vi "GTcode_v7.vi"() -> ()   [LabVIEW 2016]
uses:
  flex05-4chPascal.dll
  <vilib>/Utility/config.llb/NI_LVConfig.lvlib
  <vilib>/Utility/config.llb/Write Key (U32).vi
  <vilib>/Utility/config.llb/Read Key (U32).vi
  flex05oem8chauto100nsPASCAL_win7.dll
  <vilib>/Analysis/NI_AALBase.lvlib
  <vilib>/Utility/config.llb/Write Key (Double).vi
  <vilib>/Utility/config.llb/Read Key (I32).vi
  <vilib>/Utility/config.llb/Write Key (String).vi
  <vilib>/Utility/config.llb/Write Key (I32).vi
panel:
  out "EMG Value Text":string
  out "display number":dbl
  in  "Tab Control":T1(tab)=enum."Real Time Fitting Parameters"
  out "EMG":dbl(slide) scale=0.0..100.0
  out "mean":dbl format="%0.1e"
  out "COV":dbl format="%0.1f"
  in  "Fixed Time":bool
  in  "Detector Used":T2(ring)=enum."Det 2"
  in  "Real Time Fitting?":bool=TRUE
  out "g2":cluster{"Delay Time":sgl[], sgl[]}[](graph) caption="Normalized Correlation Function"
  out "Tau":cluster{"tmp":dbl, dbl}(graph) caption="Relative Changes of Flow"
  in  "QUIT":bool
  in  "Clear plots":bool
  in  "Baseline":bool
  in  "MARK\nMark":bool
  in  "Stop":bool
  out "Mark #":u32
  out "Trial #":u32
  out "Frame #":u32
  out "Det 8":sgl format="%.3f"
  out "Det 7":sgl format="%.3f"
  out "Det 6":sgl format="%.3f"
  out "Det 5":sgl format="%.3f"
  out "Det 4":sgl format="%.3f"
  out "Det 3":sgl format="%.3f"
  out "Det 2":sgl format="%.3f"
  out "Det 1":sgl format="%.3f"
  out "Computer Time":string="2010-1-12 23:16:10"
  in  "D1":bool
  in  "D2":bool
  in  "D3":bool
  in  "D4":bool
  in  "D5":bool
  in  "D6":bool
  in  "D7":bool
  in  "D8":bool
  out "Tau 2":T3(graph)={1.6593152555505744e-08, 3.9427894777554196e-08, 4.065716407938411e-08, 1.5135790977358522e-08, 2.4870420100428357e-08, 7.094765128107397e-08, 0.0, 4.1348620928852906e-07, 1.5886917674344795e-08, 4.0280526032721455e-08, -1.0, -1.0} caption="Blood Flow Index (cm2/s)"
  in  "Fixed # of Frames":u32=5
  out "Status":string="Quit"
  in  "Optical Switch OPEN":bool
  in  "Delay between frames(ms)":u32=500
  out "Time Left (ms)":sgl format="%.3f"
  in  "Integration Time (ms)":sgl=1000.0 min=1 max=13000 step=1
  in  "File Name (mouse#):":string="test0"
  in  "Data Save Directory:":path=path "C:/data"
  in  "ISS Lasers ON":bool
  in  "Test":bool
  in  "Right":bool
  out "R Counter":dbl format="%#_13g"
  out "saved file name":string
  in  "Left":bool
  out "L Counter":dbl format="%#_13g"
  in  "Lines":tag="Dev1/port1/line0:1, Dev1/port1/line3:7"
  in  "Delaytime(ms)":u32=200
  in  "Initialize Correlator":bool
  in  "Detector Select":enum32{"4 Detectors", "8 Detectors"}(radio)=enum."8 Detectors"
  in  "Update Time (ms)\nDO NOT CHANGE!":u32=105 min=1 max=999 step=1
  in  "Laser Input Name":refnum<visa-resource-name>="COM7"
  out "Change?":bool
  in  "Sequence Scan":bool
  out "Flow in each detector":dbl[](array[numeric])=[-1.0, -1.0, -1.0, -1.0, -1.0, -1.0, -1.0, -1.0, -1.0, -1.0, -1.0, -1.0]
  in  "Visible Averages":bool[](array[boolean])=[FALSE, FALSE, FALSE, FALSE]
  in  "Avg":bool[][](array[boolean])=[[FALSE, FALSE, FALSE, FALSE, FALSE, FALSE, FALSE, FALSE], [FALSE, FALSE, FALSE, FALSE, FALSE, FALSE, FALSE, FALSE], [FALSE, FALSE, FALSE, FALSE, FALSE, FALSE, FALSE, FALSE], [FALSE, FALSE, FALSE, FALSE, FALSE, FALSE, FALSE, FALSE]]
  in  "rho":dbl[](array[numeric])=[2.5, 2.5, 2.5, 2.5, 2.5, 2.5, 2.5, 2.5, -1.0, -1.0, -1.0, -1.0]
  in  "Other Settings":u32[](array[numeric])=[1, 120, 0, 1] caption="Flow in each detector"
  in  "Initial Guess":dbl[](array[numeric])=[1e-08, 0.5, 0.05, 10.0] caption="Flow in each detector"
  in  "UI Data Path":path=path "C:/Users/Tinggroup/Desktop/VRMuscleActivationVisualizer/LabviewFiles/Jake DCScode_GT/BiofeedbackEMGPackage/BiofeedbackData.txt"
  in  "FPS":dbl
  out "4CH?":bool
  out "Detector#":u32=1
  out "Source#":u32=1
  # "kHz"
  # "kHz"
  # "Don't Change these Parameters unless you know clearly what you are doing"
  # "ISS Triggers Setup"
  # "Channel Parameters"
  # "Step1"
  # "Line"
  # "0"
  # "1"
  # "3"
  # "4"
  # "5"
  # "6"
  # "7"
  # "*The number of lines in the list must\nmatch the number of elements in\nthe array."
  # "Step2"
  # "Line"
  # "0"
  # "1"
  # "3"
  # "4"
  # "5"
  # "6"
  # "7"
  # "Step3"
  # "Line"
  # "0"
  # "1"
  # "3"
  # "4"
  # "5"
  # "6"
  # "7"
  # "Line    Signal\n\n0           ISS Trigger (0: OFF, 1: ON)\n1           Flow Laser 1 ON/OFF (0:OFF, 1:ON)\n2           ISS Data Acquisition (0: DONE, 1: NO)\n3           ISS Laser ON/OFF (0: ON, 1: OFF)\n4           Trigger for Marks  (0: OFF, 1: ON)\n5           Flow Laser 2 ON/OFF (0:OFF, 1:ON)\n6           Reserved\n7           Reserved"
  # "Wait ISS Data Acuisition DONE Signal"
  # "Step4"
  # "Step5"
  # "Line"
  # "0"
  # "1"
  # "3"
  # "4"
  # "5"
  # "6"
  # "7"
  # "Flow Lasers Setup"
  # "FROM FRONT PANEL"
  # "Line"
  # "0"
  # "1"
  # "3"
  # "4"
  # "5"
  # "6"
  # "7"
  # "Line"
  # "0"
  # "1"
  # "3"
  # "4"
  # "5"
  # "6"
  # "7"
  # "Det 1"
  # "Det 2"
  # "Det 3"
  # "Det 4"
  # "Det 5"
  # "Det 6"
  # "Det 7"
  # "Det 8"
  # "Avg 1"
  # "Avg 2"
  # "Avg 3"
  # "Avg 4"
  # "Db"
  # "Beta"
  # "Mua"
  # "MuS'"
  # "1"
  # "2"
  # "3"
  # "4"
  # "5"
  # "6"
  # "7"
  # "8"
  # "Avg 1"
  # "Starting Pt"
  # "End Pt"
  # "Approximate"
  # "Variables"
  # "Avg 2"
  # "Avg 3"
  # "Avg 4"
  # "Source Detector  Separations"
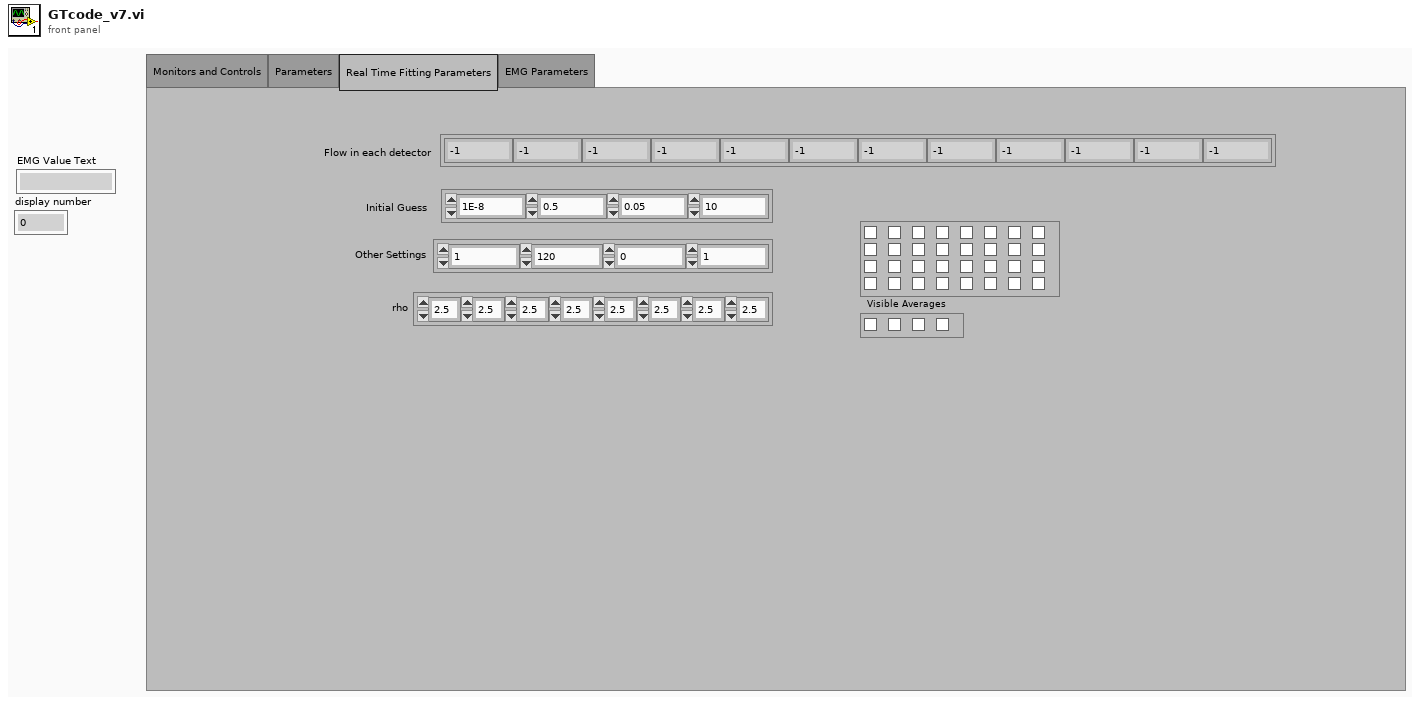
[diagram p1: front panel]
types:
  T1 = enum32{"Monitors and Controls", "Parameters", "Real Time Fitting Parameters", "EMG Parameters"}
  T2 = enum16{"Det 1", "Det 2", "Det 3", "Det 4", "Det 5", "Det 6", "Det 7", "Det 8"}
  T3 = cluster{dbl, dbl, dbl, dbl, dbl, dbl, dbl, dbl, dbl, dbl, dbl, dbl}
  T4 = enum8{"Enabled", "Disabled", "Disabled and Grayed Out"}
  T5 = cluster{dbl, dbl, dbl, dbl, dbl, dbl, dbl, dbl, dbl, dbl, dbl, dbl}[]
  T6 = typedef "NI_LVConfig.lvlib/Config Data RefNum.ctl" = refnum<k1>
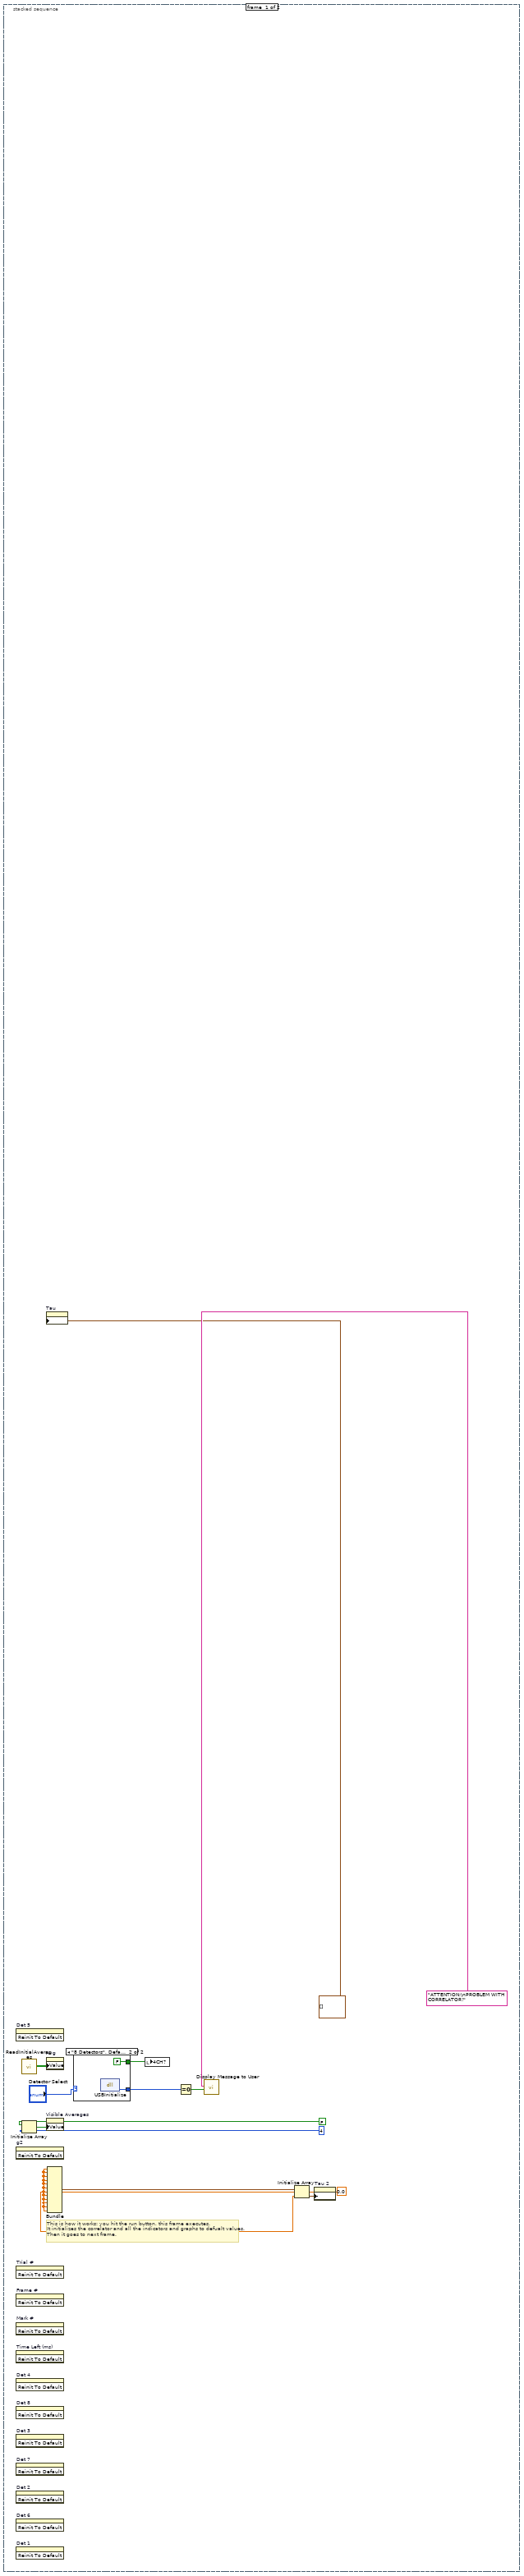
[diagram p2: hidden frame]
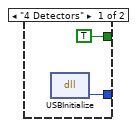
[diagram p3: hidden frame]
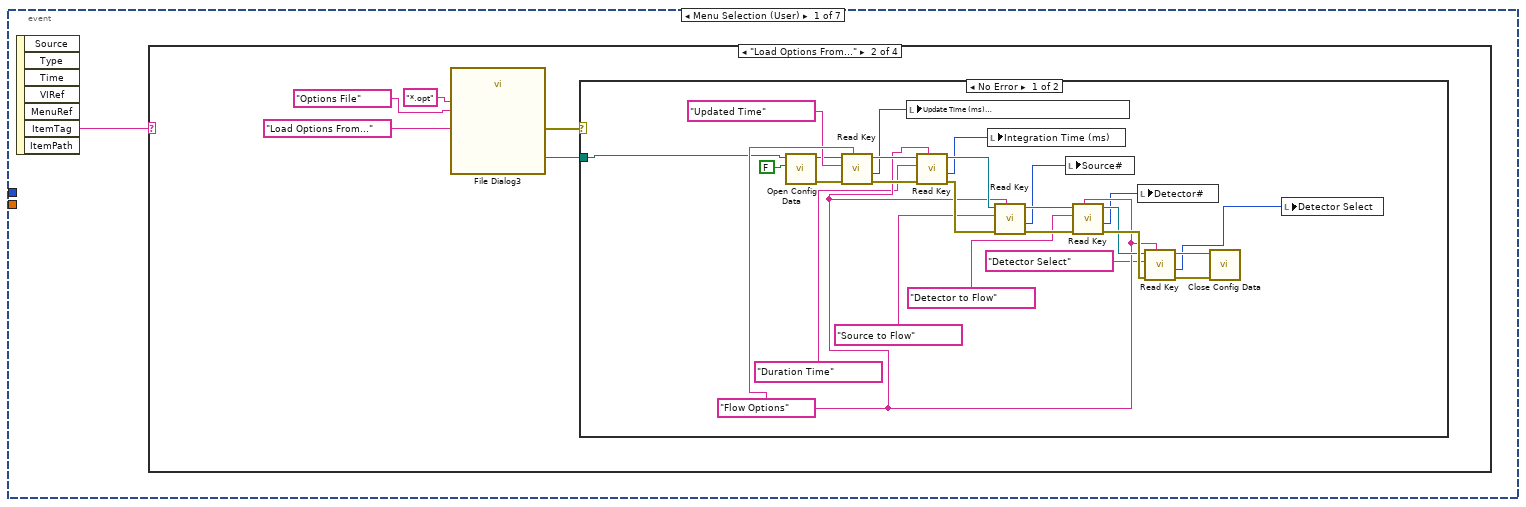
[diagram p5: hidden frame]
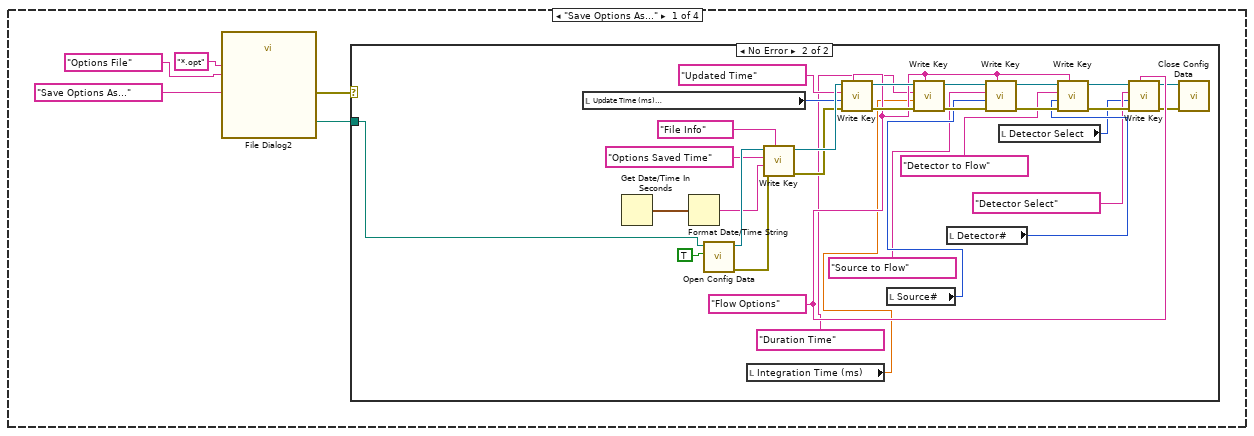
[diagram p6: hidden frame]
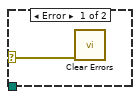
[diagram p7: hidden frame]
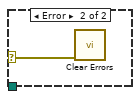
[diagram p8: hidden frame]
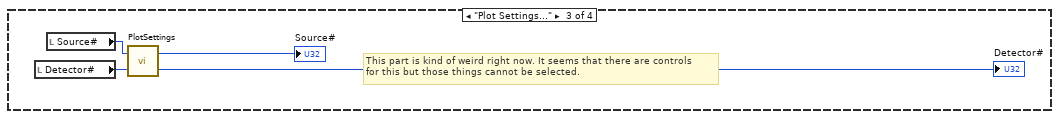
[diagram p9: hidden frame]
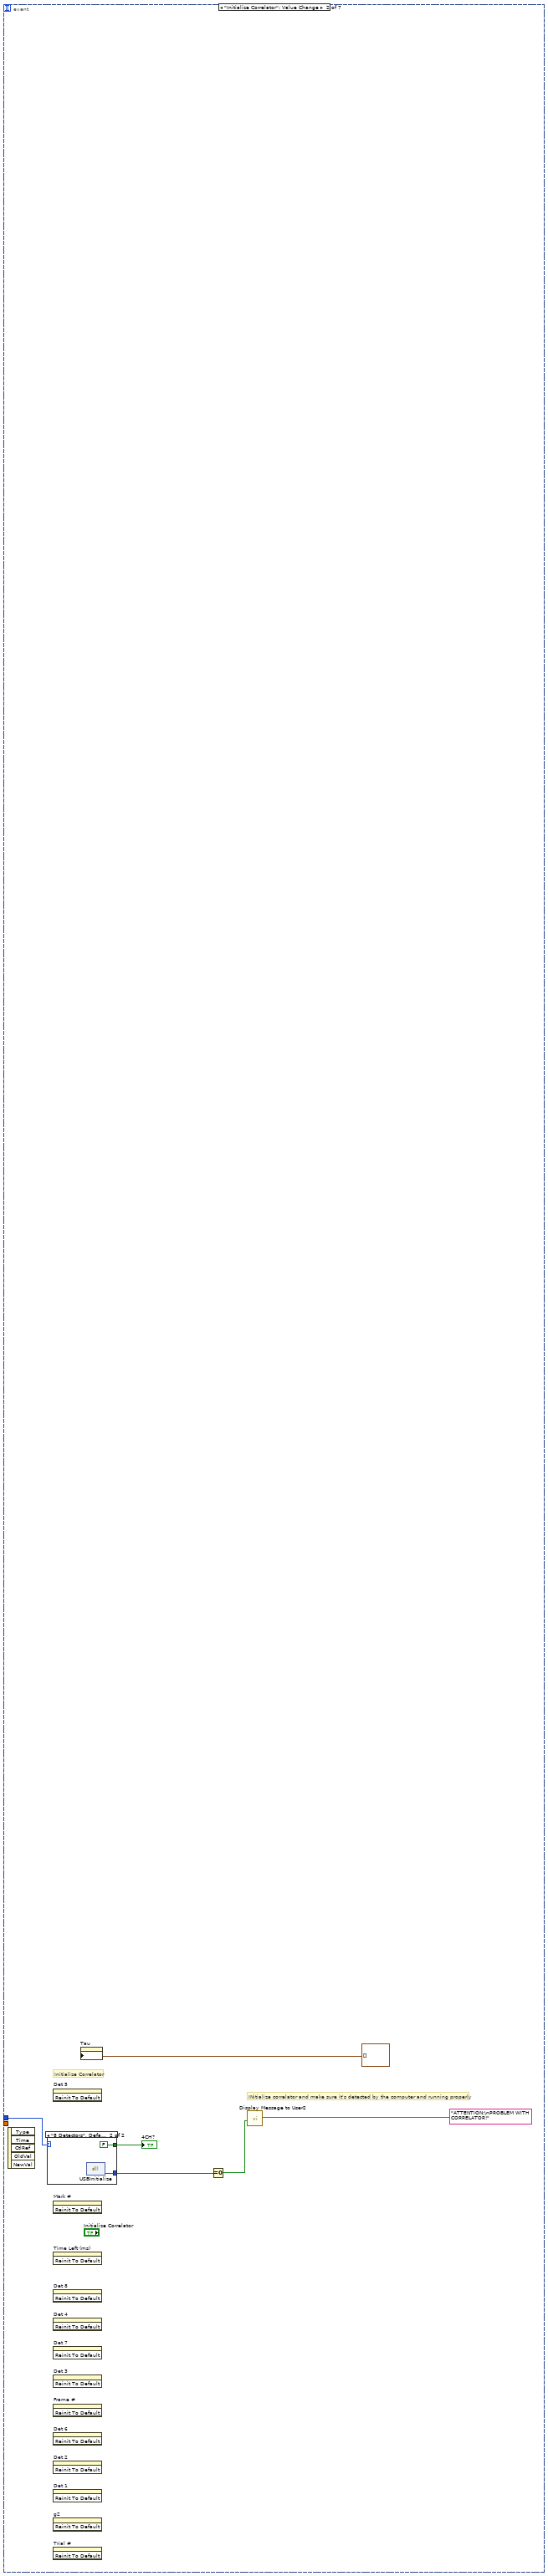
[diagram p11: hidden frame]
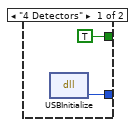
[diagram p12: hidden frame]
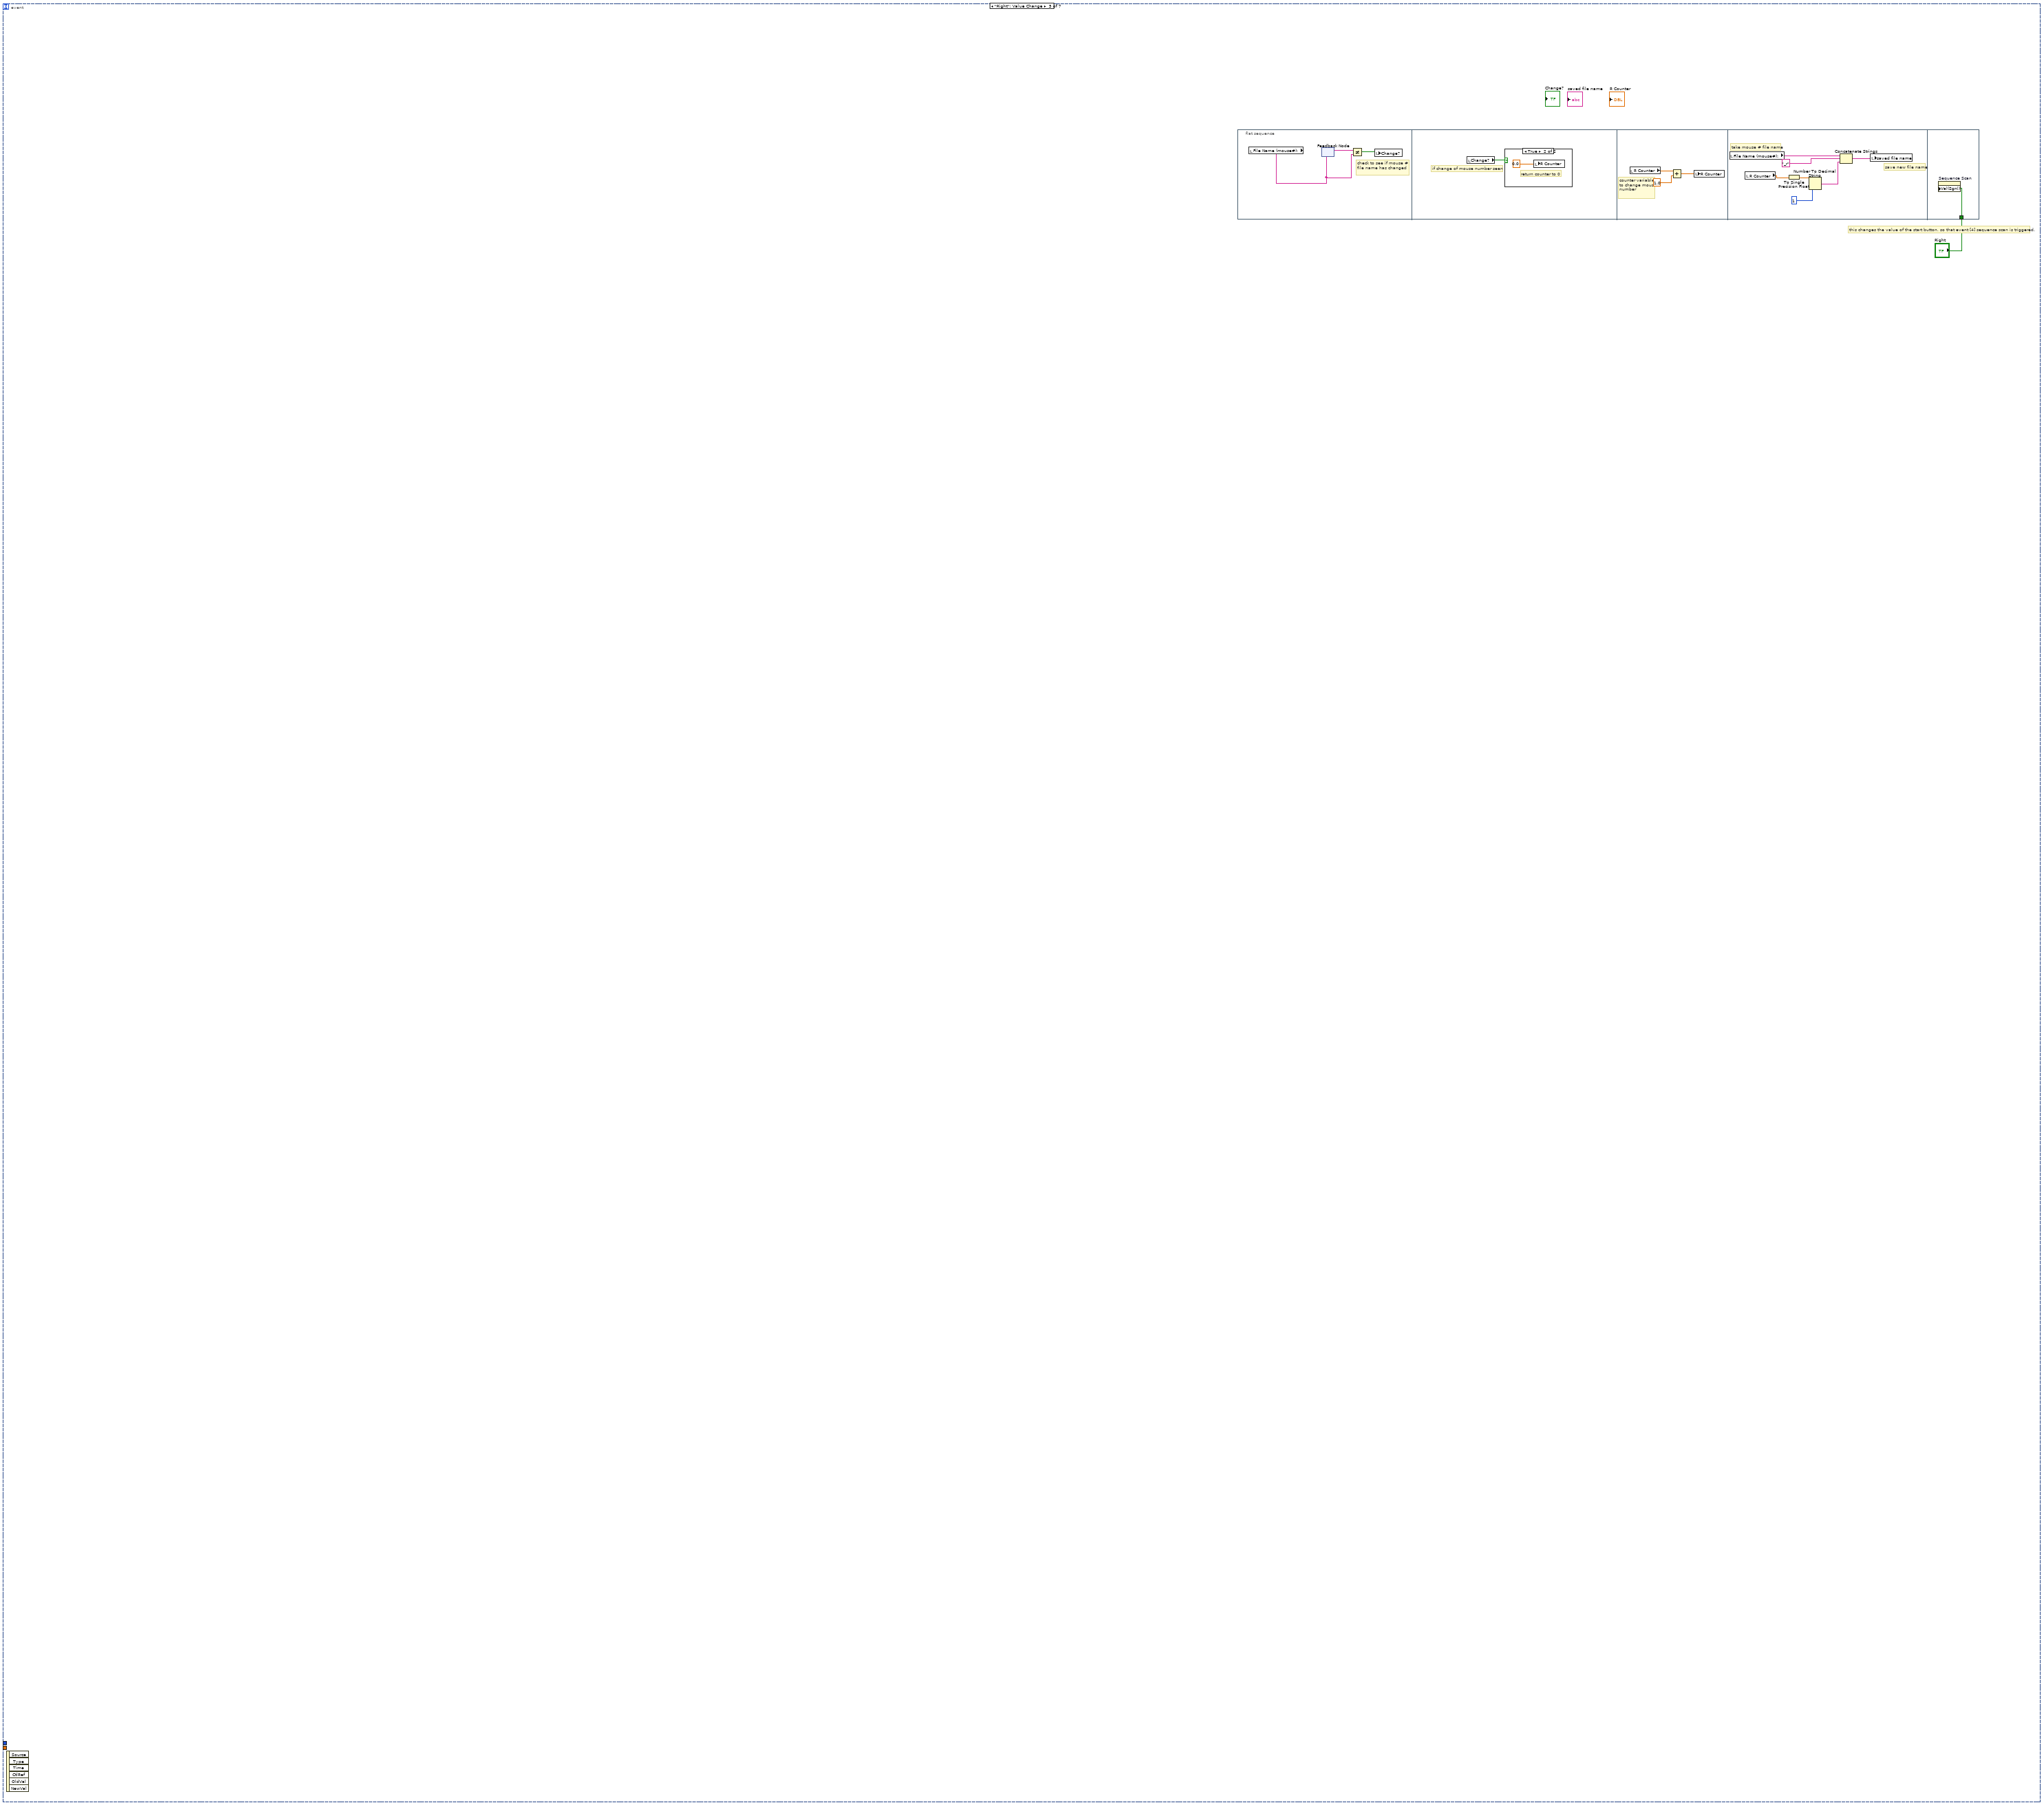
[diagram p13: hidden frame]
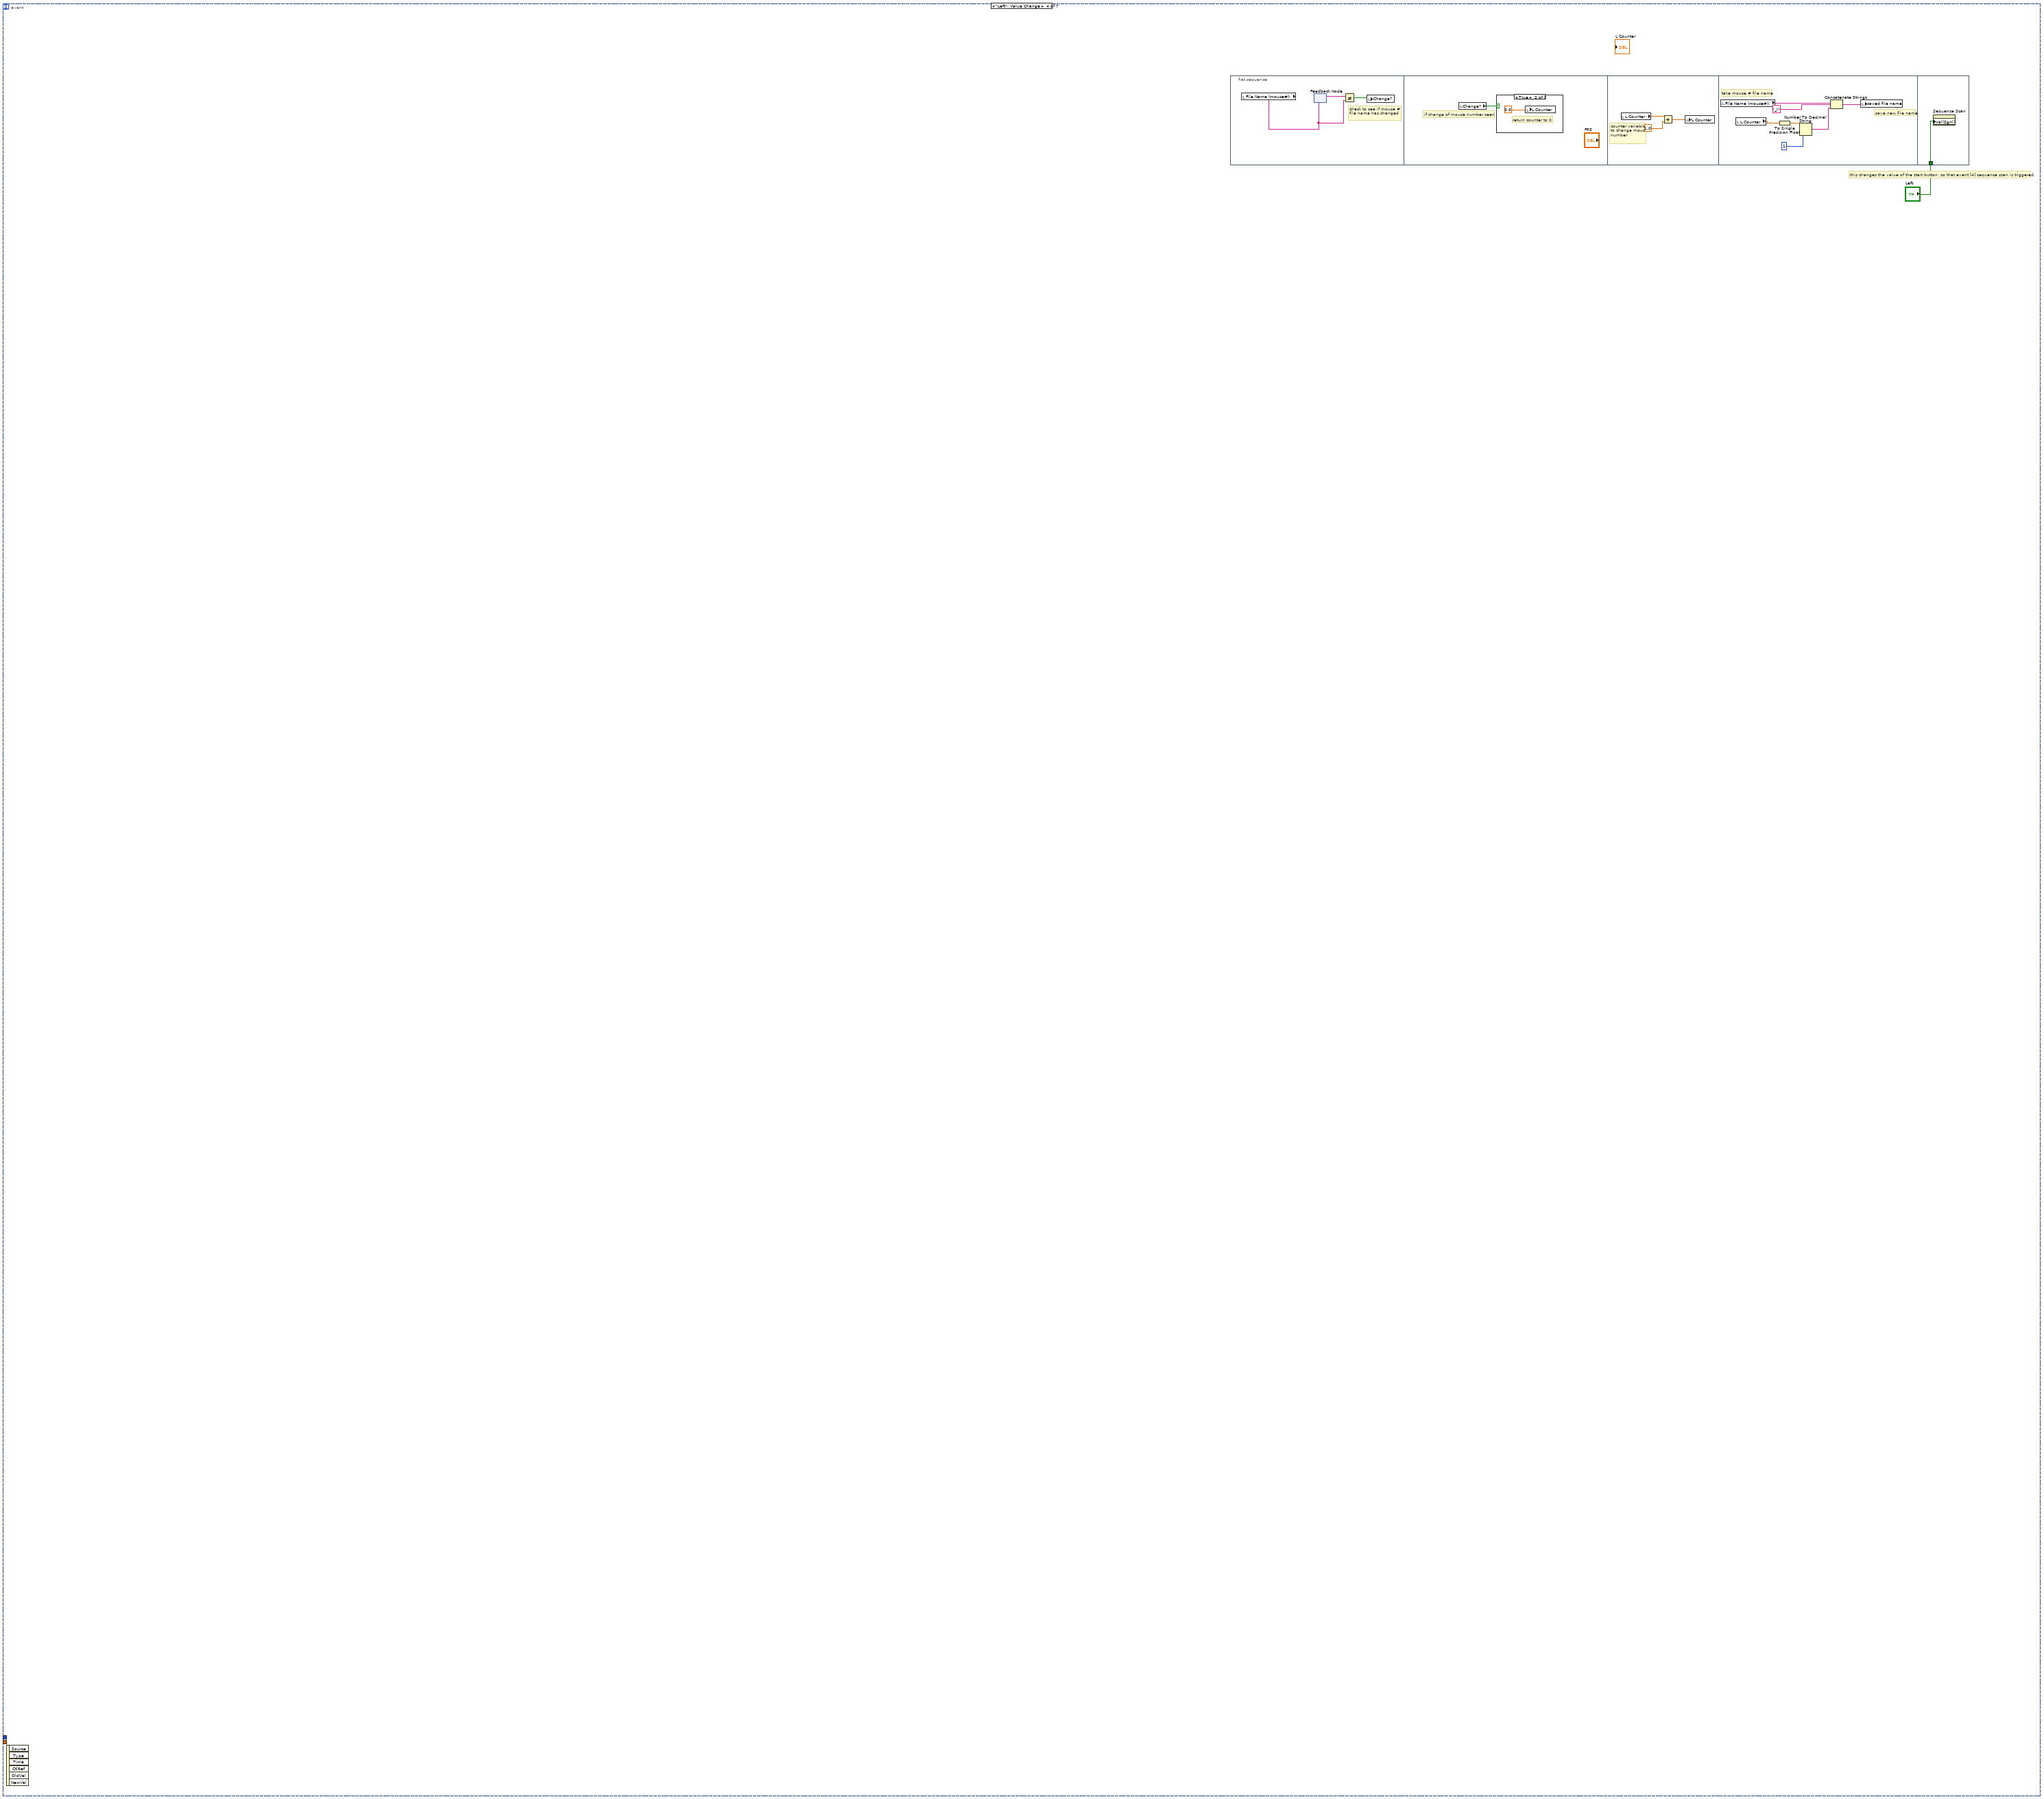
[diagram p15: hidden frame]
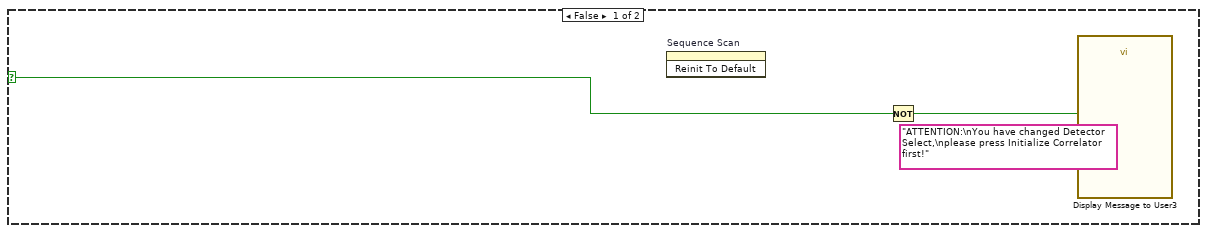
[diagram p17: hidden frame]
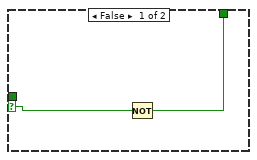
[diagram p18: hidden frame]
diagram:
  n1 = while {
    stop <- w6 stop-if-true
    n2 = local read "UI Data Path"() -> (w7:path)
    n3 = local read "Stop"() -> (w6:bool)
    n4 = Read from Text File(file (use dialog)=w7) -> (text=w5:string)  [unwired: 3 in, 3 out]
    "EMG Value Text" <- w5
    n5 = Fract/Exp String To Number(string=w5) -> (number=→"display number" →"EMG":dbl)  [unwired: 3 in, 1 out]
  }
  n6 = local read "Laser Input Name"() -> (w2:refnum<visa-resource-name>)
  n7 = call "BioFeedback7(DAQ+8-channel)SubVIToUI.vi"("UI Data Input File"="UI Data Path") -> ()  [unwired: 15 in]
  n8 = call "iBs.vi"("Laser On/Off"=FALSE, "VISA resource name"=w2) -> ()
  n9 = stacked-sequence {
    frame #0 {
      w10 = 0.0
      # "This is how it works: you hit the run button, this frame executes.\nIt initializes the correlator and all the indicators and graphs to defualt values.\nThen it goes to next frame."
      n10 = invoke on="Det 5" class="DigNum (strict)" method="Reinit To Default"() -> ()  [unwired: 3 in, 3 out]
      n11 = invoke on="g2" class="XYGraph (strict)" method="Reinit To Default"() -> ()  [unwired: 3 in, 3 out]
      n12 = invoke on="Trial #" class="DigNum (strict)" method="Reinit To Default"() -> ()  [unwired: 3 in, 3 out]
      n13 = invoke on="Frame #" class="DigNum (strict)" method="Reinit To Default"() -> ()  [unwired: 3 in, 3 out]
      n14 = invoke on="Mark #" class="DigNum (strict)" method="Reinit To Default"() -> ()  [unwired: 3 in, 3 out]
      n15 = invoke on="Time Left (ms)" class="DigNum (strict)" method="Reinit To Default"() -> ()  [unwired: 3 in, 3 out]
      n16 = invoke on="Det 4" class="DigNum (strict)" method="Reinit To Default"() -> ()  [unwired: 3 in, 3 out]
      n17 = invoke on="Det 8" class="DigNum (strict)" method="Reinit To Default"() -> ()  [unwired: 3 in, 3 out]
      n18 = invoke on="Det 3" class="DigNum (strict)" method="Reinit To Default"() -> ()  [unwired: 3 in, 3 out]
      n19 = invoke on="Det 7" class="DigNum (strict)" method="Reinit To Default"() -> ()  [unwired: 3 in, 3 out]
      n20 = invoke on="Det 2" class="DigNum (strict)" method="Reinit To Default"() -> ()  [unwired: 3 in, 3 out]
      n21 = invoke on="Det 6" class="DigNum (strict)" method="Reinit To Default"() -> ()  [unwired: 3 in, 3 out]
      n22 = invoke on="Det 1" class="DigNum (strict)" method="Reinit To Default"() -> ()  [unwired: 3 in, 3 out]
      n23 = call "ReadInitialAverages.vi"() -> ("avgOut"=w9:bool[][])  [unwired: 11 in]
      n24 = Initialize Array(FALSE, 4) -> (w8:bool[])
      n25 = property on="Tau" class="WFChart (strict)"("History Data"=cluster{"tmp":dbl, dbl}[] []) -> ()  [unwired: 2 in, 2 out]
      n26 = property on="Avg" class="Arr (strict)"("Value"=w9) -> ()  [unwired: 2 in, 2 out]
      n27 = property on="Visible Averages" class="Arr (strict)"("Value"=w8) -> ()  [unwired: 2 in, 2 out]
      n28 = Bundle(w10, w10, w10, w10, w10, w10, w10, w10, w10, w10, w10, w10) -> (w12:T3)  [unwired: 1 in]
      n29 = case shown="\"8 Detectors\", Default" "Detector Select" {
        tunnel: [w22 w24] -> w20
        tunnel: [TRUE FALSE] -> w18
        frame "4 Detectors" {
          n30 = dll-call lib="C:/Users/BUCKLEY-ADMIN/Desktop/GTcode_v6_Michelle/flex05-4chPascal.dll" fn="USBInitialize" label="InitCH4"() -> ("return type"=w22:u8)  [unwired: 3 in, 2 out]
        }
        frame "8 Detectors", Default {
          n31 = dll-call lib="C:/Users/BUCKLEY-ADMIN/Desktop/GTcode_v6_Michelle/flex05oem8chauto100nsPASCAL_win7.dll" fn="USBInitialize" label="InitCH8"() -> ("return type"=w24:u8)  [unwired: 3 in, 2 out]
        }
      }
      n32 = local write "4CH?"(w18) -> ()
      n33 = Equal To 0?(x=w20) -> (x = 0?=w19:bool)
      n34 = call "Display Message to User"("Enable"=w19, "Message"="ATTENTION:\nPROBLEM WITH CORRELATOR!") -> ()  [unwired: 8 in, 2 out]
      n35 = Initialize Array(w12, w10) -> (w11:T5)
      n36 = property on="Tau 2" class="WFChart (strict)"("History Data"=w11) -> ()  [unwired: 2 in, 2 out]
    }
    frame #1 {
      n37 = while {
        stop <- w28 stop-if-true
        # "Looks at whether using 4 or 8 ch correlator\nGenerates time points for g2 function based on correlator"
        n38 = local read "Detector Select"() -> (w26:enum32{"4 Detectors", "8 Detectors"})
        n39 = case shown="\"8 Detectors\"" w26 {
          tunnel: [_ w29] -> w25
          frame "4 Detectors", Default {
          }
          frame "8 Detectors" {
            n40 = formula code="int i,j;\nfloat DelayTime[256];\nfloat first_delay;\n\nfirst_delay = 2E-7;\n\nfor(i=0;i<16;i++)\nDelayTime[i] = (i+1)*first_delay;\nfor(j=1;j<31;j++)\n    for(i=0;i<8;i++)\n         DelayTime[i+(j-1)*8+16] = DelayTime[(j-1)*8+16+i-1]+first_delay*pow(2,j);"() -> ("DelayTime"=w29:dbl[])
          }
        }
        n41 = event shown="[4] \"Sequence Scan\": Value Change" {
          selector: _ -> [_ _ _ _ _ _ _]
          dyn-events: _ -> [_ _ _ _ _ _ _]
          timeout: 500 -> [_ _ _ _ _ _ _]
          tunnel: w25 -> [_ _ _ _ w153 _ _]
          tunnel: [_ _ _ _ _ "QUIT" _] -> w28
          tunnel: w26 -> [_ w106 _ _ w149 w637 _]
          event Menu Selection (User) {
            n42 = event-data() -> ("ItemTag"=w30:string)  [unwired: 1 in, 6 out]
            n43 = case shown="\"Load Options From...\"" w30 {
              frame "Save Options As..." {
                n44 = call "File Dialog2"("prompt"="Save Options As...", "pattern (all files)"="*.opt", "pattern label"="Options File") -> ("selected path"=w32:path, "error out"=w31:errorcluster)  [unwired: 9 in, 2 out]
                n45 = case shown="No Error" w31 {
                  selector: w31 -> [w36 _]
                  tunnel: w32 -> [_ w67]
                  frame Error {
                    n46 = call <vilib>:"Clear Errors.vi"("error in (no error)"=w36) -> ()  [unwired: 5 in, 2 out]
                  }
                  frame No Error {
                    w54 = "Flow Options"
                    n47 = local read "Update Time (ms)\nDO NOT CHANGE!"() -> (w47:u32)
                    n48 = Get Date/Time In Seconds() -> (seconds since 1Jan1904=w53:timestamp)
                    n49 = Format Date/Time String(seconds (now)=w53) -> (date/time string=w49:string)  [unwired: 2 in]
                    n50 = call <vilib>:"Open Config Data.vi"("create file if necessary (T)"=TRUE, "configuration file path"=w67) -> ("error out"=w65:errorcluster, "refnum"=w64:T6)  [unwired: 7 in, 1 out]
                    n51 = local read "Integration Time (ms)"() -> (w45:sgl)
                    n52 = call-poly <vilib>:"Write Key.vi"("section"="File Info", "error in (no error)"=w65, "value"=w49, "key"="Options Saved Time", "refnum"=w64) -> ("error out"=w51:errorcluster, "refnum out"=w52:T6)  [unwired: 4 in, 1 out]
                    n53 = call-poly <vilib>:"Write Key.vi"("section"=w54, "error in (no error)"=w51, "value"=w47, "key"="Updated Time", "refnum"=w52) -> ("error out"=w63:errorcluster, "refnum out"=w62:T6)  [unwired: 4 in, 1 out]
                    n54 = local read "Source#"() -> (w44:u32)
                    n55 = call-poly <vilib>:"Write Key.vi"("section"=w54, "error in (no error)"=w63, "value"=w45, "key"="Duration Time", "refnum"=w62) -> ("error out"=w58:errorcluster, "refnum out"=w59:T6)  [unwired: 4 in, 1 out]
                    n56 = local read "Detector#"() -> (w41:u32)
                    n57 = call-poly <vilib>:"Write Key.vi"("section"=w54, "error in (no error)"=w58, "value"=w44, "key"="Source to Flow", "refnum"=w59) -> ("error out"=w60:errorcluster, "refnum out"=w61:T6)  [unwired: 4 in, 1 out]
                    n58 = local read "Detector Select"() -> (w39:enum32{"4 Detectors", "8 Detectors"})
                    n59 = call-poly <vilib>:"Write Key.vi"("section"=w54, "error in (no error)"=w60, "value"=w41, "key"="Detector to Flow", "refnum"=w61) -> ("error out"=w57:errorcluster, "refnum out"=w56:T6)  [unwired: 4 in, 1 out]
                    n60 = call-poly <vilib>:"Write Key.vi"("section"=w54, "error in (no error)"=w57, "value"=w39, "key"="Detector Select", "refnum"=w56) -> ("error out"=w37:errorcluster, "refnum out"=w38:T6)  [unwired: 4 in, 1 out]
                    n61 = call <vilib>:"Close Config Data.vi"("error in (no error)"=w37, "refnum"=w38) -> ()  [unwired: 8 in, 2 out]
                  }
                }
              }
              frame "Load Options From..." {
                n62 = call "File Dialog3"("prompt"="Load Options From...", "pattern (all files)"="*.opt", "pattern label"="Options File") -> ("selected path"=w69:path, "error out"=w68:errorcluster)  [unwired: 9 in, 2 out]
                n63 = case shown="No Error" w68 {
                  selector: w68 -> [_ w98]
                  tunnel: w69 -> [w73 _]
                  frame No Error {
                    w88 = "Flow Options"
                    n64 = call <vilib>:"Open Config Data.vi"("create file if necessary (T)"=FALSE, "configuration file path"=w73) -> ("error out"=w80:errorcluster, "refnum"=w79:T6)  [unwired: 7 in, 1 out]
                    n65 = call-poly <vilib>:"Read Key.vi"("section"=w88, "error in (no error)"=w80, "key"="Updated Time", "refnum"=w79) -> ("error out"=w96:errorcluster, "value"=w78:u32, "refnum out"=w95:T6)  [unwired: 4 in, 1 out]
                    n66 = local write "Update Time (ms)\nDO NOT CHANGE!"(w78) -> ()
                    n67 = call-poly <vilib>:"Read Key.vi"("section"=w88, "error in (no error)"=w96, "key"="Duration Time", "refnum"=w95) -> ("error out"=w91:errorcluster, "value"=w77:i32, "refnum out"=w92:T6)  [unwired: 4 in, 1 out]
                    n68 = local write "Integration Time (ms)"(w77) -> ()
                    n69 = call-poly <vilib>:"Read Key.vi"("section"=w88, "error in (no error)"=w91, "key"="Source to Flow", "refnum"=w92) -> ("error out"=w93:errorcluster, "value"=w74:u32, "refnum out"=w94:T6)  [unwired: 4 in, 1 out]
                    n70 = local write "Source#"(w74) -> ()
                    n71 = call-poly <vilib>:"Read Key.vi"("section"=w88, "error in (no error)"=w93, "key"="Detector to Flow", "refnum"=w94) -> ("error out"=w90:errorcluster, "value"=w75:u32, "refnum out"=w89:T6)  [unwired: 4 in, 1 out]
                    n72 = local write "Detector#"(w75) -> ()
                    n73 = call-poly <vilib>:"Read Key.vi"("section"=w88, "error in (no error)"=w90, "key"="Detector Select", "refnum"=w89) -> ("error out"=w81:errorcluster, "value"=w76:u32, "refnum out"=w82:T6)  [unwired: 4 in, 1 out]
                    n74 = call <vilib>:"Close Config Data.vi"("error in (no error)"=w81, "refnum"=w82) -> ()  [unwired: 8 in, 2 out]
                    n75 = local write "Detector Select"(w76) -> ()
                  }
                  frame Error {
                    n76 = call <vilib>:"Clear Errors.vi"("error in (no error)"=w98) -> ()  [unwired: 5 in, 2 out]
                  }
                }
              }
              frame "Plot Settings..." {
                # "This part is kind of weird right now. It seems that there are controls\nfor this but those things cannot be selected."
                n77 = local read "Detector#"() -> (w100:u32)
                n78 = local read "Source#"() -> (w101:u32)
                n79 = call "PlotSettings.vi"("Detectorin"=w100, "Sourcein"=w101) -> ("Detector#"=→"Detector#":u32, "Source#"=→"Source#":u32)
              }
              frame Default {
              }
            }
          }
          event "Initialize Correlator": Value Change {
            # "INitialize correlator and make sure it's detected by the computer and running properly"
            # "Initialize Correlator"
            n80 = event-data() -> ()  [unwired: 1 in, 5 out]
            n81 = case shown="\"8 Detectors\", Default" w106 {
              tunnel: [w110 w112] -> w108
              tunnel: [TRUE FALSE] -> w105
              frame "4 Detectors" {
                n82 = dll-call lib="C:/Users/BUCKLEY-ADMIN/Desktop/GTcode_v6_Michelle/flex05-4chPascal.dll" fn="USBInitialize" label="InitCH4"() -> ("return type"=w110:u8)  [unwired: 3 in, 2 out]
              }
              frame "8 Detectors", Default {
                n83 = dll-call lib="C:/Users/BUCKLEY-ADMIN/Desktop/GTcode_v6_Michelle/flex05oem8chauto100nsPASCAL_win7.dll" fn="USBInitialize" label="InitCH8"() -> ("return type"=w112:u8)  [unwired: 3 in, 2 out]
              }
            }
            "4CH?" <- w105
            n84 = invoke on="Det 5" class="DigNum (strict)" method="Reinit To Default"() -> ()  [unwired: 3 in, 3 out]
            n85 = invoke on="Mark #" class="DigNum (strict)" method="Reinit To Default"() -> ()  [unwired: 3 in, 3 out]
            n86 = invoke on="Time Left (ms)" class="DigNum (strict)" method="Reinit To Default"() -> ()  [unwired: 3 in, 3 out]
            n87 = invoke on="Det 8" class="DigNum (strict)" method="Reinit To Default"() -> ()  [unwired: 3 in, 3 out]
            n88 = invoke on="Det 4" class="DigNum (strict)" method="Reinit To Default"() -> ()  [unwired: 3 in, 3 out]
            n89 = invoke on="Det 7" class="DigNum (strict)" method="Reinit To Default"() -> ()  [unwired: 3 in, 3 out]
            n90 = invoke on="Det 3" class="DigNum (strict)" method="Reinit To Default"() -> ()  [unwired: 3 in, 3 out]
            n91 = invoke on="Frame #" class="DigNum (strict)" method="Reinit To Default"() -> ()  [unwired: 3 in, 3 out]
            n92 = invoke on="Det 6" class="DigNum (strict)" method="Reinit To Default"() -> ()  [unwired: 3 in, 3 out]
            n93 = invoke on="Det 2" class="DigNum (strict)" method="Reinit To Default"() -> ()  [unwired: 3 in, 3 out]
            n94 = invoke on="Det 1" class="DigNum (strict)" method="Reinit To Default"() -> ()  [unwired: 3 in, 3 out]
            n95 = invoke on="g2" class="XYGraph (strict)" method="Reinit To Default"() -> ()  [unwired: 3 in, 3 out]
            n96 = invoke on="Trial #" class="DigNum (strict)" method="Reinit To Default"() -> ()  [unwired: 3 in, 3 out]
            n97 = property on="Tau" class="WFChart (strict)"("History Data"=cluster{"tmp":dbl, dbl}[] []) -> ()  [unwired: 2 in, 2 out]
            n98 = Equal To 0?(x=w108) -> (x = 0?=w107:bool)
            n99 = call "Display Message to User2"("Enable"=w107, "Message"="ATTENTION:\nPROBLEM WITH CORRELATOR!") -> ()  [unwired: 8 in, 2 out]
          }
          event "Right": Value Change {
            # "this changes the value of the start button, so that event [4] sequence scan is triggered."
            n100 = event-data() -> ()  [unwired: 1 in, 6 out]
            n101 = flat-sequence {
              tunnel: "Right" -> [w129]
              frame #0 {
                # "check to see if mouse # file name has changed"
                n102 = local read "File Name (mouse#):"() -> (w115:string)
                n103 = feedback #1() -> (w116:string)  [unwired: 1 in]
                n104 = feedback-in #1(w115) -> ()
                n105 = Not Equal?(x=w116, y=w115) -> (x != y?=w114:bool)
                n106 = local write "Change?"(w114) -> ()
              }
              frame #1 {
                # "if change of mouse number seen"
                n107 = local read "Change?"() -> (w117:bool)
                n108 = case shown="True" w117 {
                  frame False {
                  }
                  frame True {
                    # "return counter to 0"
                    n109 = local write "R Counter"(0.0) -> ()
                  }
                }
              }
              frame #2 {
                # "counter variable to change mouse number"
                n110 = local read "R Counter"() -> (w120:dbl)
                n111 = Add(x=w120, y=1.0) -> (x+y=w119:dbl)
                n112 = local write "R Counter"(w119) -> ()
              }
              frame #3 {
                # "save new file name"
                # "take mouse # file name"
                n113 = local read "File Name (mouse#):"() -> (w127:string)
                n114 = local read "R Counter"() -> (w122:dbl)
                n115 = To Single Precision Float(number=w122) -> (single precision float=w123:sgl)
                n116 = Number To Decimal String(number=w123, width (-)=1) -> (decimal integer string=w125:string)
                n117 = Concatenate Strings(w127, "_r", w125) -> (w126:string)
                n118 = local write "saved file name"(w126) -> ()
              }
              frame #4 {
                n119 = property on="Sequence Scan" class="Bool (strict)"("Val(Sgnl)"=w129) -> ()  [unwired: 2 in, 2 out]
              }
            }
          }
          event "Left": Value Change {
            # "this changes the value of the start button, so that event [4] sequence scan is triggered."
            n120 = event-data() -> ()  [unwired: 1 in, 6 out]
            n121 = flat-sequence {
              tunnel: "Left" -> [w146]
              frame #0 {
                # "check to see if mouse # file name has changed"
                n122 = local read "File Name (mouse#):"() -> (w132:string)
                n123 = feedback #2() -> (w133:string)  [unwired: 1 in]
                n124 = feedback-in #2(w132) -> ()
                n125 = Not Equal?(x=w133, y=w132) -> (x != y?=w131:bool)
                n126 = local write "Change?"(w131) -> ()
              }
              frame #1 {
                # "if change of mouse number seen"
                n127 = local read "Change?"() -> (w134:bool)
                n128 = case shown="True" w134 {
                  frame False {
                  }
                  frame True {
                    # "return counter to 0"
                    n129 = local write "L Counter"(0.0) -> ()
                  }
                }
              }
              frame #2 {
                # "counter variable to change mouse number"
                n130 = local read "L Counter"() -> (w137:dbl)
                n131 = Add(x=w137, y=1.0) -> (x+y=w136:dbl)
                n132 = local write "L Counter"(w136) -> ()
              }
              frame #3 {
                # "save new file name"
                # "take mouse # file name"
                n133 = local read "File Name (mouse#):"() -> (w144:string)
                n134 = local read "L Counter"() -> (w139:dbl)
                n135 = To Single Precision Float(number=w139) -> (single precision float=w140:sgl)
                n136 = Number To Decimal String(number=w140, width (-)=1) -> (decimal integer string=w142:string)
                n137 = Concatenate Strings(w144, "_l", w142) -> (w143:string)
                n138 = local write "saved file name"(w143) -> ()
              }
              frame #4 {
                n139 = property on="Sequence Scan" class="Bool (strict)"("Val(Sgnl)"=w146) -> ()  [unwired: 2 in, 2 out]
              }
            }
          }
          event "Sequence Scan": Value Change {
            # "Initialize Baseline"
            n140 = event-data() -> ()  [unwired: 1 in, 6 out]
            n141 = case shown="\"8 Detectors\", Default" w149 {
              tunnel: [w632 w633] -> w148
              frame "4 Detectors" {
                n142 = local read "4CH?"() -> (w632:bool)
              }
              frame "8 Detectors", Default {
                # "Select whether using 4 or 8ch correlator"
                n143 = local read "4CH?"() -> (w634:bool)
                n144 = Not(x=w634) -> (.not. x?=w633:bool)
              }
            }
            n145 = case shown="True" w148 {
              selector: w148 -> [w155 _]
              tunnel: w153 -> [_ w169]
              tunnel: w149 -> [_ w170]
              tunnel: sgl 1.0 -> [_ w168]
              frame False {
                n146 = invoke on="Sequence Scan" class="Bool (strict)" method="Reinit To Default"() -> ()  [unwired: 3 in, 3 out]
                n147 = Not(x=w155) -> (.not. x?=w154:bool)
                n148 = call "Display Message to User3"("Enable"=w154, "Message"="ATTENTION:\nYou have changed Detector Select,\nplease press Initialize Correlator first!") -> ()  [unwired: 8 in, 2 out]
              }
              frame True {
                # "This part pauses and alerts user that test function is on. If test function is accepted then code runs but data is not saved (no timestamp either)."
                # "This checks for if the file already exists in the directory using the timing file. \n*If YES, then we don't do anything to the lasers. We just display message and wait for the user to input a new name and press sequence again.\n*If NO, then we proceed as per normal."
                n149 = local read "File Name (mouse#):"() -> (w164:string)
                n150 = case shown="True" "Test" {
                  selector: "Test" -> [w172 _]
                  tunnel: "Test" -> [_ w174]
                  tunnel: [w171 w173] -> w157
                  frame False {
                    n151 = Not(x=w172) -> (.not. x?=w171:bool)
                  }
                  frame True {
                    n152 = call "Test ON"("Enable"=w174) -> ("No - STOP"=w175:bool, "OK"=w173:bool)  [unwired: 15 in, 2 out]
                    n153 = local write "Stop"(w175) -> ()
                  }
                }
                n154 = local read "Data Save Directory:"() -> (w163:path)
                n155 = Concatenate Strings(w164, "_TIMING", ".dat") -> (w166:string)
                n156 = Build Path(base path=w163, name or relative path=w166) -> (appended path=w162:path)
                n157 = call <vilib>:"Check if File or Folder Exists.vi"("path"=w162) -> ("file or folder exists?"=w159:bool)  [unwired: 8 in, 2 out]
                n158 = Not(x=w159) -> (.not. x?=w161:bool)
                n159 = Not And(1:w157, 2:w161) -> (0:w160:bool)
                n160 = case shown="False" w160 {
                  tunnel: w170 -> [w189 _]
                  tunnel: w169 -> [w188 _]
                  tunnel: w168 -> [w187 _]
                  frame False {
                    # "Turn relay on so that Optical switch is open and LED indicator is ON"
                    # "When the START button is pressed, the ISS lasers turn off"
                    n161 = local read "Test"() -> (w176:bool)
                    n162 = case shown="False" w176 {
                      frame False {
                        # "This bit stores the time stamp."
                        n163 = local read "saved file name"() -> (w190:string)
                        n164 = Get Date/Time In Seconds() -> (seconds since 1Jan1904=w192:timestamp)
                        n165 = local read "Data Save Directory:"() -> (w191:path)
                        n166 = Format Date/Time String(seconds (now)=w192) -> (date/time string=w198:string)  [unwired: 2 in]
                        n167 = Concatenate Strings(w190, "_TIMING", ".dat") -> (w195:string)
                        n168 = Build Path(base path=w191, name or relative path=w195) -> (appended path=w194:path)
                        n169 = Write to Text File(file (use dialog)=w194, text=w198) -> (refnum out=w197:refnum<file>, error out=w196:errorcluster)  [unwired: 2 in, 1 out]
                        n170 = Close File(refnum=w197, error in=w196) -> ()  [unwired: 2 out]
                      }
                      frame True {
                      }
                    }
                    n171 = Build Array(TRUE, TRUE) -> (w186:bool[])
                    n172 = Build Array(FALSE) -> (w183:bool[])
                    n173 = local read "Fixed # of Frames"() -> (w181:u32)
                    n174 = call "DAQ Assistant"("data"=w186) -> ()  [unwired: 17 in, 2 out]
                    n175 = call "DAQ Assistant7"("data"=w183) -> ()  [unwired: 17 in, 2 out]
                    n176 = Initialize Array "Initialize Array"(nan, w181) -> (w179:dbl[])
                    n177 = while {
                      tunnel: w189 -> [w233]
                      tunnel: w188 -> [w232]
                      tunnel: w187 -> [_]
                      shift-right: [w204] -> _
                      shift-left: w179 -> [w205]
                      stop <- w206 stop-if-true
                      # "Only runs Real Time Fitting if \nReal Time Fitting box is checked \nand test function is off."
                      # "After testing is complete, turn off the lasers and\nreset  the buttons."
                      n178 = for {
                        N: 1 -> [_]
                        tunnel: w232 -> [w274]
                        tunnel: w233 -> [w273]
                        tunnel: [w270] -> w206
                        tunnel: [w269] -> w230
                        tunnel: [w267] -> w210
                        tunnel: [w266] -> w209
                        tunnel: [w265] -> w208
                        # "The logic here may look funny but it works elegantly. No matter if you choose \"Use Both Lasers\", the AND output is always\nfalse the first time these two boxes run since Laser 1 Value is always false, and the default is to use flow laser 1.\nBUT, the trick is if you chose \"Use Both Laser\" This big for loop is gonna run twice, the second time it runs, \nthe laser 1 value is TRUE because it is set to TRUE by the second box when the big for loop ran the first time. Now, when\nthe output of AND is true, ISS laser no longer runs. Only flow laser two is turned on and we execute the for loop to the right."
                        # "These two boxes take care of the flow chart.\nIt turn on ISS laser first, then triggers it and turn it off.\nIf ISS data is ready, then we go on to flow lase."
                        # "This loop may seem useless but it acts as a block. \nThis block does all the data collection, plotting and writing the data\nto file"
                        n179 = case shown="\"8 Detectors\", Default" w273 {
                          selector: w273 -> [w630 w631]
                          tunnel: [w630 w631] -> w271
                          frame "4 Detectors" {
                            n180 = dll-call lib="C:/Users/BUCKLEY-ADMIN/Desktop/GTcode_v6_Michelle/flex05-4chPascal.dll" fn="USBStart" label="StartCH4"() -> ()  [unwired: 4 in, 2 out]
                          }
                          frame "8 Detectors", Default {
                            n181 = dll-call lib="C:/Users/BUCKLEY-ADMIN/Desktop/GTcode_v6_Michelle/flex05oem8chauto100nsPASCAL_win7.dll" fn="USBStart" label="StartCH8"() -> ()  [unwired: 4 in, 2 out]
                          }
                        }
                        n182 = for {
                          N: 1 -> [_]
                          tunnel: w274 -> [w296]
                          tunnel: [w280] -> w270
                          tunnel: w271 -> [w285]
                          tunnel: [w288] -> w269
                          tunnel: "MARK\nMark" -> [w287]
                          tunnel: [w286] -> w267
                          tunnel: [w277] -> w266
                          tunnel: [w284] -> w265
                          w297 = FALSE
                          w306 = u8 2
                          # "Only saves data if\ntest function is off."
                          # "If Fixed # Frames check box is selected,\ncode will run for # of frames specified on \nfront panel and then call Stop button"
                          # "This for loop here acts as a block as well. It takes the relative \nflow data from UpdateData.vi and plot the data on the graph.\nWhen \"Baseline\" is selected,  the data point goes to 1. When\n\"Mark\" is selected, a point at positive infinity is plotted and a\nvertical line joining the point and the x axis if displayed."
                          n183 = while {
                            tunnel: [w486] -> w305
                            tunnel: [w456] -> w304
                            tunnel: [w457] -> w303
                            tunnel: [w460] -> w280
                            tunnel: [w487] -> w302
                            tunnel: w296 -> [w489]
                            tunnel: w285 -> [w462]
                            stop <- w491 stop-if-true
                            # "D4 Tail Alarm"
                            # "D2 Tail Alarm"
                            # "D8 Tail Alarm"
                            # "D7 Tail Alarm"
                            # "D6 Tail Alarm"
                            # "D5 Tail Alarm"
                            # "D3 Tail Alarm"
                            # "D1 Tail Alarm"
                            # "When press STOP, turn off DCS laser LED indicator is OFF"
                            n184 = Not(x="D4") -> (.not. x?=w475:bool)
                            n185 = Not(x="D8") -> (.not. x?=w471:bool)
                            n186 = Not(x="D5") -> (.not. x?=w474:bool)
                            n187 = Not(x="D1") -> (.not. x?=w478:bool)
                            n188 = Not(x="D6") -> (.not. x?=w473:bool)
                            n189 = Not(x="D2") -> (.not. x?=w463:bool)
                            n190 = Not(x="D7") -> (.not. x?=w472:bool)
                            n191 = Not(x="D3") -> (.not. x?=w476:bool)
                            n192 = case shown="True" "Stop" {
                              selector: "Stop" -> [w530 w536]
                              tunnel: [w530 w533] -> w460
                              frame False {
                              }
                              frame True {
                                n193 = call "Prompt User for Input"("Enable"=w536) -> ("Yes"=w533:bool)  [unwired: 17 in, 1 out]
                                n194 = Build Array(w533, FALSE) -> (w535:bool[])
                                n195 = call "DAQ Assistant2"("data"=w535) -> ()  [unwired: 17 in, 2 out]
                                n196 = local read "Laser Input Name"() -> (w531:refnum<visa-resource-name>)
                                n197 = call "iBs.vi"("Laser On/Off"=FALSE, "VISA resource name"=w531) -> ()
                              }
                            }
                            n198 = case shown="True" "Clear plots" {
                              frame False {
                              }
                              frame True {
                                n199 = invoke on="g2" class="XYGraph (strict)" method="Reinit To Default"() -> ()  [unwired: 3 in, 3 out]
                              }
                            }
                            n200 = case shown="False" w475 {
                              selector: w475 -> [w577 w582]
                              frame False {
                                n201 = property on="Tau 2" class="WFChart (strict)"("Active Plot"=u32 3) -> (error out=w579:errorcluster)  [unwired: 2 in, 1 out]
                                n202 = property on="g2" class="XYGraph (strict)"("Active Plot"=u32 3) -> (error out=w580:errorcluster)  [unwired: 2 in, 1 out]
                                n203 = property on="g2" class="XYGraph (strict)"(error in=w580, "Plot.Visible?"=w577) -> ()  [unwired: 1 in, 2 out]
                                n204 = property on="Tau 2" class="WFChart (strict)"(error in=w579, "Plot.Visible?"=w577) -> ()  [unwired: 1 in, 2 out]
                              }
                              frame True {
                                n205 = property on="Tau 2" class="WFChart (strict)"("Active Plot"=u32 3) -> (error out=w583:errorcluster)  [unwired: 2 in, 1 out]
                                n206 = property on="Tau 2" class="WFChart (strict)"(error in=w583, "Plot.Visible?"=w582) -> ()  [unwired: 1 in, 2 out]
                                n207 = property on="g2" class="XYGraph (strict)"("Active Plot"=u32 3) -> (error out=w585:errorcluster)  [unwired: 2 in, 1 out]
                                n208 = property on="g2" class="XYGraph (strict)"(error in=w585, "Plot.Visible?"=w582) -> ()  [unwired: 1 in, 2 out]
                              }
                            }
                            n209 = case shown="False" w471 {
                              selector: w471 -> [w537 w542]
                              frame False {
                                n210 = property on="Tau 2" class="WFChart (strict)"("Active Plot"=u32 7) -> (error out=w538:errorcluster)  [unwired: 2 in, 1 out]
                                n211 = property on="g2" class="XYGraph (strict)"("Active Plot"=u32 7) -> (error out=w540:errorcluster)  [unwired: 2 in, 1 out]
                                n212 = property on="g2" class="XYGraph (strict)"(error in=w540, "Plot.Visible?"=w537) -> ()  [unwired: 1 in, 2 out]
                                n213 = property on="Tau 2" class="WFChart (strict)"(error in=w538, "Plot.Visible?"=w537) -> ()  [unwired: 1 in, 2 out]
                              }
                              frame True {
                                n214 = property on="Tau 2" class="WFChart (strict)"("Active Plot"=u32 7) -> (error out=w544:errorcluster)  [unwired: 2 in, 1 out]
                                n215 = property on="Tau 2" class="WFChart (strict)"(error in=w544, "Plot.Visible?"=w542) -> ()  [unwired: 1 in, 2 out]
                                n216 = property on="g2" class="XYGraph (strict)"("Active Plot"=u32 7) -> (error out=w545:errorcluster)  [unwired: 2 in, 1 out]
                                n217 = property on="g2" class="XYGraph (strict)"(error in=w545, "Plot.Visible?"=w542) -> ()  [unwired: 1 in, 2 out]
                              }
                            }
                            n218 = case shown="False" w474 {
                              selector: w474 -> [w567 w572]
                              frame False {
                                n219 = property on="Tau 2" class="WFChart (strict)"("Active Plot"=u32 4) -> (error out=w569:errorcluster)  [unwired: 2 in, 1 out]
                                n220 = property on="g2" class="XYGraph (strict)"("Active Plot"=u32 4) -> (error out=w570:errorcluster)  [unwired: 2 in, 1 out]
                                n221 = property on="g2" class="XYGraph (strict)"(error in=w570, "Plot.Visible?"=w567) -> ()  [unwired: 1 in, 2 out]
                                n222 = property on="Tau 2" class="WFChart (strict)"(error in=w569, "Plot.Visible?"=w567) -> ()  [unwired: 1 in, 2 out]
                              }
                              frame True {
                                n223 = property on="Tau 2" class="WFChart (strict)"("Active Plot"=u32 4) -> (error out=w574:errorcluster)  [unwired: 2 in, 1 out]
                                n224 = property on="Tau 2" class="WFChart (strict)"(error in=w574, "Plot.Visible?"=w572) -> ()  [unwired: 1 in, 2 out]
                                n225 = property on="g2" class="XYGraph (strict)"("Active Plot"=u32 4) -> (error out=w575:errorcluster)  [unwired: 2 in, 1 out]
                                n226 = property on="g2" class="XYGraph (strict)"(error in=w575, "Plot.Visible?"=w572) -> ()  [unwired: 1 in, 2 out]
                              }
                            }
                            n227 = case shown="False" w478 {
                              selector: w478 -> [w607 w612]
                              frame False {
                                n228 = property on="Tau 2" class="WFChart (strict)"("Active Plot"=u32 0) -> (error out=w608:errorcluster)  [unwired: 2 in, 1 out]
                                n229 = property on="g2" class="XYGraph (strict)"("Active Plot"=u32 0) -> (error out=w610:errorcluster)  [unwired: 2 in, 1 out]
                                n230 = property on="g2" class="XYGraph (strict)"(error in=w610, "Plot.Visible?"=w607) -> ()  [unwired: 1 in, 2 out]
                                n231 = property on="Tau 2" class="WFChart (strict)"(error in=w608, "Plot.Visible?"=w607) -> ()  [unwired: 1 in, 2 out]
                              }
                              frame True {
                                n232 = property on="Tau 2" class="WFChart (strict)"("Active Plot"=u32 0) -> (error out=w614:errorcluster)  [unwired: 2 in, 1 out]
                                n233 = property on="Tau 2" class="WFChart (strict)"(error in=w614, "Plot.Visible?"=w612) -> ()  [unwired: 1 in, 2 out]
                                n234 = property on="g2" class="XYGraph (strict)"("Active Plot"=u32 0) -> (error out=w615:errorcluster)  [unwired: 2 in, 1 out]
                                n235 = property on="g2" class="XYGraph (strict)"(error in=w615, "Plot.Visible?"=w612) -> ()  [unwired: 1 in, 2 out]
                              }
                            }
                            n236 = case shown="False" w473 {
                              selector: w473 -> [w557 w562]
                              frame False {
                                n237 = property on="Tau 2" class="WFChart (strict)"("Active Plot"=u32 5) -> (error out=w559:errorcluster)  [unwired: 2 in, 1 out]
                                n238 = property on="g2" class="XYGraph (strict)"("Active Plot"=u32 5) -> (error out=w560:errorcluster)  [unwired: 2 in, 1 out]
                                n239 = property on="g2" class="XYGraph (strict)"(error in=w560, "Plot.Visible?"=w557) -> ()  [unwired: 1 in, 2 out]
                                n240 = property on="Tau 2" class="WFChart (strict)"(error in=w559, "Plot.Visible?"=w557) -> ()  [unwired: 1 in, 2 out]
                              }
                              frame True {
                                n241 = property on="Tau 2" class="WFChart (strict)"("Active Plot"=u32 5) -> (error out=w563:errorcluster)  [unwired: 2 in, 1 out]
                                n242 = property on="Tau 2" class="WFChart (strict)"(error in=w563, "Plot.Visible?"=w562) -> ()  [unwired: 1 in, 2 out]
                                n243 = property on="g2" class="XYGraph (strict)"("Active Plot"=u32 5) -> (error out=w565:errorcluster)  [unwired: 2 in, 1 out]
                                n244 = property on="g2" class="XYGraph (strict)"(error in=w565, "Plot.Visible?"=w562) -> ()  [unwired: 1 in, 2 out]
                              }
                            }
                            n245 = case shown="False" w463 {
                              selector: w463 -> [w597 w602]
                              frame False {
                                n246 = property on="Tau 2" class="WFChart (strict)"("Active Plot"=u32 1) -> (error out=w599:errorcluster)  [unwired: 2 in, 1 out]
                                n247 = property on="g2" class="XYGraph (strict)"("Active Plot"=u32 1) -> (error out=w600:errorcluster)  [unwired: 2 in, 1 out]
                                n248 = property on="g2" class="XYGraph (strict)"(error in=w600, "Plot.Visible?"=w597) -> ()  [unwired: 1 in, 2 out]
                                n249 = property on="Tau 2" class="WFChart (strict)"(error in=w599, "Plot.Visible?"=w597) -> ()  [unwired: 1 in, 2 out]
                              }
                              frame True {
                                n250 = property on="Tau 2" class="WFChart (strict)"("Active Plot"=u32 1) -> (error out=w604:errorcluster)  [unwired: 2 in, 1 out]
                                n251 = property on="Tau 2" class="WFChart (strict)"(error in=w604, "Plot.Visible?"=w602) -> ()  [unwired: 1 in, 2 out]
                                n252 = property on="g2" class="XYGraph (strict)"("Active Plot"=u32 1) -> (error out=w605:errorcluster)  [unwired: 2 in, 1 out]
                                n253 = property on="g2" class="XYGraph (strict)"(error in=w605, "Plot.Visible?"=w602) -> ()  [unwired: 1 in, 2 out]
                              }
                            }
                            n254 = case shown="False" w472 {
                              selector: w472 -> [w547 w552]
                              frame False {
                                n255 = property on="Tau 2" class="WFChart (strict)"("Active Plot"=u32 6) -> (error out=w549:errorcluster)  [unwired: 2 in, 1 out]
                                n256 = property on="g2" class="XYGraph (strict)"("Active Plot"=u32 6) -> (error out=w550:errorcluster)  [unwired: 2 in, 1 out]
                                n257 = property on="g2" class="XYGraph (strict)"(error in=w550, "Plot.Visible?"=w547) -> ()  [unwired: 1 in, 2 out]
                                n258 = property on="Tau 2" class="WFChart (strict)"(error in=w549, "Plot.Visible?"=w547) -> ()  [unwired: 1 in, 2 out]
                              }
                              frame True {
                                n259 = property on="Tau 2" class="WFChart (strict)"("Active Plot"=u32 6) -> (error out=w553:errorcluster)  [unwired: 2 in, 1 out]
                                n260 = property on="Tau 2" class="WFChart (strict)"(error in=w553, "Plot.Visible?"=w552) -> ()  [unwired: 1 in, 2 out]
                                n261 = property on="g2" class="XYGraph (strict)"("Active Plot"=u32 6) -> (error out=w555:errorcluster)  [unwired: 2 in, 1 out]
                                n262 = property on="g2" class="XYGraph (strict)"(error in=w555, "Plot.Visible?"=w552) -> ()  [unwired: 1 in, 2 out]
                              }
                            }
                            n263 = case shown="False" w476 {
                              selector: w476 -> [w587 w592]
                              frame False {
                                n264 = property on="Tau 2" class="WFChart (strict)"("Active Plot"=u32 2) -> (error out=w588:errorcluster)  [unwired: 2 in, 1 out]
                                n265 = property on="g2" class="XYGraph (strict)"("Active Plot"=u32 2) -> (error out=w590:errorcluster)  [unwired: 2 in, 1 out]
                                n266 = property on="g2" class="XYGraph (strict)"(error in=w590, "Plot.Visible?"=w587) -> ()  [unwired: 1 in, 2 out]
                                n267 = property on="Tau 2" class="WFChart (strict)"(error in=w588, "Plot.Visible?"=w587) -> ()  [unwired: 1 in, 2 out]
                              }
                              frame True {
                                n268 = property on="Tau 2" class="WFChart (strict)"("Active Plot"=u32 2) -> (error out=w594:errorcluster)  [unwired: 2 in, 1 out]
                                n269 = property on="Tau 2" class="WFChart (strict)"(error in=w594, "Plot.Visible?"=w592) -> ()  [unwired: 1 in, 2 out]
                                n270 = property on="g2" class="XYGraph (strict)"("Active Plot"=u32 2) -> (error out=w595:errorcluster)  [unwired: 2 in, 1 out]
                                n271 = property on="g2" class="XYGraph (strict)"(error in=w595, "Plot.Visible?"=w592) -> ()  [unwired: 1 in, 2 out]
                              }
                            }
                            n272 = Wait (ms)(milliseconds to wait="Update Time (ms)\nDO NOT CHANGE!") -> ()  [unwired: 1 out]
                            n273 = call "UpdateData.vi"("Duration Time (ms)"="Integration Time (ms)", "Detector Select"=w462, "Delay Time"=w489) -> ("Elapsed Time(s)"=w490:sgl, "Intensity Array"=w488:sgl[], "Tau Array"=w487:sgl[], "mean"=w452:dbl, "mean 8"=w432:dbl, "mean 2"=w401:dbl, "mean 7"=w433:dbl, "mean 3"=w437:dbl, "Intensity data"=w486:string, "g2 Display"=→"g2":cluster{"Delay Time":sgl[], sgl[]}[], "mean 4"=w436:dbl, "mean 5"=w435:dbl, "mean 6"=w434:dbl, "tau data"=w456:string, "g2 data"=w457:string)  [unwired: 2 in]
                            n274 = Multiply(x=sgl 1000.0, y=w490) -> (x*y=w494:sgl)
                            n275 = Less?(x=w452, y=1.005) -> (x < y?=w431:bool)
                            n276 = Less?(x=w401, y=1.005) -> (x < y?=w385:bool)
                            n277 = Less?(x=w437, y=1.005) -> (x < y?=w384:bool)
                            n278 = Less?(x=w436, y=1.005) -> (x < y?=w381:bool)
                            n279 = Less?(x=w435, y=1.005) -> (x < y?=w379:bool)
                            n280 = Less?(x=w434, y=1.005) -> (x < y?=w377:bool)
                            n281 = Less?(x=w433, y=1.005) -> (x < y?=w375:bool)
                            n282 = Less?(x=w432, y=1.005) -> (x < y?=w373:bool)
                            n283 = Index Array(array=w488, index #1=0, index #2=1, index #3=2, index #4=3, index #5=4, index #6=5, index #7=6, index #8=7) -> (element #1=w429:sgl, element #2=w408:sgl, element #3=w407:sgl, element #4=w406:sgl, element #5=w405:sgl, element #6=w404:sgl, element #7=w403:sgl, element #8=w402:sgl)
                            "Det 7" <- w403
                            "Det 6" <- w404
                            "Det 5" <- w405
                            "Det 4" <- w406
                            "Det 3" <- w407
                            "Det 2" <- w408
                            "Det 1" <- w429
                            "Det 8" <- w402
                            n284 = Subtract(x="Integration Time (ms)", y=w494) -> (x-y=w492:sgl)
                            "Time Left (ms)" <- w492
                            n285 = Greater?(x=w452, y=0.98) -> (0:w430:bool)
                            n286 = Greater?(x=w436, y=0.98) -> (0:w382:bool)
                            n287 = Greater?(x=w434, y=0.98) -> (0:w378:bool)
                            n288 = Greater?(x=w432, y=0.98) -> (0:w374:bool)
                            n289 = Greater Or Equal?(x=w429, y=sgl 2.0) -> (x >= y?=w426:bool)
                            n290 = Greater Or Equal?(x=w408, y=sgl 2.0) -> (x >= y?=w372:bool)
                            n291 = Greater Or Equal?(x=w407, y=sgl 2.0) -> (x >= y?=w370:bool)
                            n292 = Greater Or Equal?(x=w406, y=sgl 2.0) -> (x >= y?=w368:bool)
                            n293 = Greater Or Equal?(x=w405, y=sgl 2.0) -> (x >= y?=w366:bool)
                            n294 = Greater Or Equal?(x=w404, y=sgl 2.0) -> (x >= y?=w364:bool)
                            n295 = Less Or Equal?(x=w429, y=sgl 1000.0) -> (x <= y?=w425:bool)
                            n296 = Less Or Equal?(x=w408, y=sgl 1000.0) -> (x <= y?=w371:bool)
                            n297 = Less Or Equal?(x=w407, y=sgl 1000.0) -> (x <= y?=w369:bool)
                            n298 = Less Or Equal?(x=w406, y=sgl 1000.0) -> (x <= y?=w367:bool)
                            n299 = Less Or Equal?(x=w405, y=sgl 1000.0) -> (x <= y?=w365:bool)
                            n300 = Less Or Equal?(x=w404, y=sgl 1000.0) -> (x <= y?=w363:bool)
                            n301 = Less Or Equal?(x=w403, y=sgl 1000.0) -> (x <= y?=w361:bool)
                            n302 = Less Or Equal?(x=w402, y=sgl 1000.0) -> (x <= y?=w359:bool)
                            n303 = Greater Or Equal?(x=w403, y=sgl 2.0) -> (x >= y?=w362:bool)
                            n304 = Greater Or Equal?(x=w402, y=sgl 2.0) -> (x >= y?=w360:bool)
                            n305 = Greater?(x=w401, y=0.98) -> (0:w386:bool)
                            n306 = Greater?(x=w437, y=0.98) -> (0:w383:bool)
                            n307 = Greater?(x=w435, y=0.98) -> (0:w380:bool)
                            n308 = Greater?(x=w433, y=0.98) -> (0:w376:bool)
                            n309 = Build Array(w431, w430, w426, w425) -> (w424:bool[])
                            n310 = Build Array(w386, w385, w372, w371) -> (w400:bool[])
                            n311 = Build Array(w384, w383, w370, w369) -> (w399:bool[])
                            n312 = Build Array(w382, w381, w368, w367) -> (w398:bool[])
                            n313 = Build Array(w380, w379, w366, w365) -> (w397:bool[])
                            n314 = Build Array(w378, w377, w364, w363) -> (w396:bool[])
                            n315 = Build Array(w376, w375, w362, w361) -> (w395:bool[])
                            n316 = Build Array(w374, w373, w360, w359) -> (w394:bool[])
                            n317 = And Array Elements(Boolean array=w424) -> (logical AND=w423:bool)
                            n318 = And Array Elements(Boolean array=w400) -> (logical AND=w387:bool)
                            n319 = And Array Elements(Boolean array=w399) -> (logical AND=w388:bool)
                            n320 = And Array Elements(Boolean array=w398) -> (logical AND=w389:bool)
                            n321 = And Array Elements(Boolean array=w397) -> (logical AND=w390:bool)
                            n322 = And Array Elements(Boolean array=w396) -> (logical AND=w391:bool)
                            n323 = And Array Elements(Boolean array=w395) -> (logical AND=w392:bool)
                            n324 = And Array Elements(Boolean array=w394) -> (logical AND=w393:bool)
                            n325 = Less Or Equal To 0?(x=w492) -> (x <= 0?=w493:bool)
                            n326 = case shown="True" w423 {
                              frame False {
                                n327 = control-ref of="Det 1"() -> (w526:refnum<vi>)
                                n328 = property on="Property Node" class="Digital (strict)"(reference=w526, "DisabledEnum"=T4."Disabled and Grayed Out" ("Disabled")) -> ()  [unwired: 1 in, 2 out]
                              }
                              frame True {
                                n329 = control-ref of="Det 1"() -> (w528:refnum<vi>)
                                n330 = property on="Property Node" class="Digital (strict)"(reference=w528, "DisabledEnum"=T4."Enabled" ("Disabled")) -> ()  [unwired: 1 in, 2 out]
                              }
                            }
                            n331 = case shown="True" w387 {
                              frame False {
                                n332 = control-ref of="Det 2"() -> (w522:refnum<vi>)
                                n333 = property on="Property Node" class="Digital (strict)"(reference=w522, "DisabledEnum"=T4."Disabled and Grayed Out" ("Disabled")) -> ()  [unwired: 1 in, 2 out]
                              }
                              frame True {
                                n334 = control-ref of="Det 2"() -> (w524:refnum<vi>)
                                n335 = property on="Property Node" class="Digital (strict)"(reference=w524, "DisabledEnum"=T4."Enabled" ("Disabled")) -> ()  [unwired: 1 in, 2 out]
                              }
                            }
                            n336 = case shown="True" w388 {
                              frame False {
                                n337 = control-ref of="Det 3"() -> (w518:refnum<vi>)
                                n338 = property on="Property Node" class="Digital (strict)"(reference=w518, "DisabledEnum"=T4."Disabled and Grayed Out" ("Disabled")) -> ()  [unwired: 1 in, 2 out]
                              }
                              frame True {
                                n339 = control-ref of="Det 3"() -> (w520:refnum<vi>)
                                n340 = property on="Property Node" class="Digital (strict)"(reference=w520, "DisabledEnum"=T4."Enabled" ("Disabled")) -> ()  [unwired: 1 in, 2 out]
                              }
                            }
                            n341 = case shown="True" w389 {
                              frame False {
                                n342 = control-ref of="Det 4"() -> (w514:refnum<vi>)
                                n343 = property on="Property Node" class="Digital (strict)"(reference=w514, "DisabledEnum"=T4."Disabled and Grayed Out" ("Disabled")) -> ()  [unwired: 1 in, 2 out]
                              }
                              frame True {
                                n344 = control-ref of="Det 4"() -> (w516:refnum<vi>)
                                n345 = property on="Property Node" class="Digital (strict)"(reference=w516, "DisabledEnum"=T4."Enabled" ("Disabled")) -> ()  [unwired: 1 in, 2 out]
                              }
                            }
                            n346 = case shown="True" w390 {
                              frame False {
                                n347 = control-ref of="Det 5"() -> (w510:refnum<vi>)
                                n348 = property on="Property Node" class="Digital (strict)"(reference=w510, "DisabledEnum"=T4."Disabled and Grayed Out" ("Disabled")) -> ()  [unwired: 1 in, 2 out]
                              }
                              frame True {
                                n349 = control-ref of="Det 5"() -> (w512:refnum<vi>)
                                n350 = property on="Property Node" class="Digital (strict)"(reference=w512, "DisabledEnum"=T4."Enabled" ("Disabled")) -> ()  [unwired: 1 in, 2 out]
                              }
                            }
                            n351 = case shown="False" w391 {
                              frame False {
                                n352 = control-ref of="Det 6"() -> (w506:refnum<vi>)
                                n353 = property on="Property Node" class="Digital (strict)"(reference=w506, "DisabledEnum"=T4."Disabled and Grayed Out" ("Disabled")) -> ()  [unwired: 1 in, 2 out]
                              }
                              frame True {
                                n354 = control-ref of="Det 6"() -> (w508:refnum<vi>)
                                n355 = property on="Property Node" class="Digital (strict)"(reference=w508, "DisabledEnum"=T4."Enabled" ("Disabled")) -> ()  [unwired: 1 in, 2 out]
                              }
                            }
                            n356 = case shown="True" w392 {
                              frame False {
                                n357 = control-ref of="Det 7"() -> (w502:refnum<vi>)
                                n358 = property on="Property Node" class="Digital (strict)"(reference=w502, "DisabledEnum"=T4."Disabled and Grayed Out" ("Disabled")) -> ()  [unwired: 1 in, 2 out]
                              }
                              frame True {
                                n359 = control-ref of="Det 7"() -> (w504:refnum<vi>)
                                n360 = property on="Property Node" class="Digital (strict)"(reference=w504, "DisabledEnum"=T4."Enabled" ("Disabled")) -> ()  [unwired: 1 in, 2 out]
                              }
                            }
                            n361 = case shown="True" w393 {
                              frame False {
                                n362 = control-ref of="Det 8"() -> (w498:refnum<vi>)
                                n363 = property on="Property Node" class="Digital (strict)"(reference=w498, "DisabledEnum"=T4."Disabled and Grayed Out" ("Disabled")) -> ()  [unwired: 1 in, 2 out]
                              }
                              frame True {
                                n364 = control-ref of="Det 8"() -> (w500:refnum<vi>)
                                n365 = property on="Property Node" class="Digital (strict)"(reference=w500, "DisabledEnum"=T4."Enabled" ("Disabled")) -> ()  [unwired: 1 in, 2 out]
                              }
                            }
                            n366 = Or(x=w460, y=w493) -> (x .or. y?=w491:bool)
                            n367 = case shown="True" w491 {
                              tunnel: w462 -> [w617 _]
                              frame True {
                                n368 = case shown="\"8 Detectors\", Default" w617 {
                                frame "4 Detectors" {
                                n369 = dll-call lib="C:/Users/BUCKLEY-ADMIN/Desktop/GTcode_v6_Michelle/flex05-4chPascal.dll" fn="USBStop" label="StopCH4"() -> ()  [unwired: 4 in, 2 out]
                                }
                                frame "8 Detectors", Default {
                                n370 = dll-call lib="C:/Users/BUCKLEY-ADMIN/Desktop/GTcode_v6_Michelle/flex05oem8chauto100nsPASCAL_win7.dll" fn="USBStop" label="StopCH8"() -> ()  [unwired: 4 in, 2 out]
                                }
                                }
                              }
                              frame False {
                              }
                            }
                          }
                          n371 = Current VI's Menubar() -> (w299:refnum<k9>)
                          n372 = local read "Trial #"() -> (w292:u32)
                          n373 = property on="QUIT" class="Bool"("Disabled"=w306) -> ()  [unwired: 2 in, 2 out]
                          n374 = Set Menu Item Info(7:"File", 9:w297, 11:w299) -> (3:w298:refnum<k9>)  [unwired: 4 in, 1 out]
                          n375 = Increment(x=w292) -> (x+1=w291:u32)
                          n376 = property on="Sequence Scan" class="Bool (strict)"("Disabled"=w306) -> ()  [unwired: 2 in, 2 out]
                          n377 = property on="Update Time (ms)\nDO NOT CHANGE!" class="DigNum (strict)"("Disabled"=w306) -> ()  [unwired: 2 in, 2 out]
                          n378 = property on="Integration Time (ms)" class="DigNum (strict)"("Disabled"=w306) -> ()  [unwired: 2 in, 2 out]
                          n379 = property on="Detector Select" class="RadioBtnsControl (strict)"("Disabled"=w306) -> ()  [unwired: 2 in, 2 out]
                          n380 = property on="Initialize Correlator" class="Bool"("Disabled"=w306) -> ()  [unwired: 2 in, 2 out]
                          n381 = local write "Trial #"(w291) -> ()
                          n382 = Set Menu Item Info(7:"Options", 9:w297, 11:w298) -> ()  [unwired: 4 in, 2 out]
                          n383 = case shown="\"Det 2\"" "Detector Used" {
                            tunnel: [1 2 3 4 5 6 7 8] -> w294
                            frame "Det 1", Default {
                            }
                            frame "Det 2" {
                            }
                            frame "Det 3" {
                            }
                            frame "Det 4" {
                            }
                            frame "Det 5" {
                            }
                            frame "Det 6" {
                            }
                            frame "Det 7" {
                            }
                            frame "Det 8" {
                            }
                          }
                          n384 = for {
                            N: 1 -> [_]
                            tunnel: w302 -> [w347]
                            tunnel: [w350] -> w295
                            tunnel: w294 -> [w349]
                            tunnel: w287 -> [w340]
                            n385 = case shown="True" w340 {
                              tunnel: [u32 0 w356] -> w350
                              frame False {
                              }
                              frame True {
                                n386 = local write "Trial #"(u32 0) -> ()
                                n387 = local read "Mark #"() -> (w358:u32)
                                n388 = Increment(x=w358) -> (x+1=w356:u32)
                                n389 = local write "Mark #"(w356) -> ()
                              }
                            }
                            n390 = Index Array(array=w347, index=w349) -> (element=w348:sgl)
                            n391 = Boolean To (0,1)(Boolean="Baseline") -> (0, 1=w352:i16)
                            n392 = case shown="False" w340 {
                              tunnel: [0.0 w354] -> w344
                              tunnel: inf -> [_ w354]
                              frame False {
                              }
                              frame True {
                              }
                            }
                            n393 = feedback #3() -> (w345:sgl)  [unwired: 1 in]
                            n394 = formula code="if(Tau==0) Tau=Tau+0.001;\nif(T==1) baselineflow=Tau;\n\ntmp=baselineflow/Tau;"("Tau"=w348, "T"=w352, "baselineflow"=w345) -> ("tmp"=w342:dbl, "baselineflow"=w346:sgl)
                            n395 = feedback-in #3(w346) -> ()
                            n396 = Bundle("tmp"=w342, w344) -> (→"Tau":cluster{"tmp":dbl, dbl})  [unwired: 1 in]
                          }
                          n397 = property on="Frame #" class="DigNum (strict)"() -> ("Value"=w278:u32)  [unwired: 2 in, 2 out]
                          n398 = case shown="True" "Fixed Time" {
                            tunnel: w278 -> [w328 w331]
                            tunnel: [w328 w331] -> w277
                            frame False {
                            }
                            frame True {
                              n399 = Less Or Equal?(x="Fixed # of Frames", y=w331) -> (x <= y?=w329:bool)
                              n400 = local write "Stop"(w329) -> ()
                            }
                          }
                          n401 = case shown="\"8 Detectors\", Default" w285 {
                            tunnel: w295 -> [w625 w629]
                            tunnel: [w626 w628] -> w312
                            tunnel: [4 8] -> w284
                            frame "4 Detectors" {
                              n402 = Build Array(w625, w625, w625, w625, w625) -> (w626:u32[])
                            }
                            frame "8 Detectors", Default {
                              n403 = Build Array(w629, w629, w629, w629, w629, w629, w629, w629, w629) -> (w628:u32[])
                            }
                          }
                          n404 = case shown="\"8 Detectors\", Default" w285 {
                            tunnel: ["%Duration\tID1\t\tID2\t\tID3\t\tID4\n" "%Duration\tID1\t\tID2\t\tID3\t\tID4\t\tID5\t\tID6\t\tID7\t\tID8\n"] -> w309
                            tunnel: ["%Tau\t\tTau1\t\tTau2\t\tTau3\t\tTau4\n" "%Tau\t\tTau1\t\tTau2\t\tTau3\t\tTau4\t\tTau5\t\tTau6\t\tTau7\t\tTau8\n"] -> w308
                            tunnel: ["%Delaytime\tD1\t\tD2\t\tD3\t\tD4\n" "%Delaytime\tD1\t\tD2\t\tD3\t\tD4\t\tD5\t\tD6\t\tD7\t\tD8\n"] -> w307
                            frame "4 Detectors" {
                            }
                            frame "8 Detectors", Default {
                            }
                          }
                          n405 = local read "saved file name"() -> (w275:string)
                          n406 = Increment(x=w277) -> (x+1=w279:u32)
                          n407 = Number To Decimal String(number=w277) -> (decimal integer string=w313:string)  [unwired: 1 in]
                          n408 = local write "Frame #"(w279) -> ()
                          n409 = Get Date/Time In Seconds() -> (seconds since 1Jan1904=w321:timestamp)
                          n410 = Array To Spreadsheet String(array=w312, 3:"%d") -> (spreadsheet string=w310:string)  [unwired: 1 in]
                          n411 = Format Date/Time String(seconds (now)=w321) -> (date/time string=w318:string)  [unwired: 2 in]
                          "Computer Time" <- w318
                          n412 = Concatenate Strings(w275, "_flow_", w313, ".dat") -> (w282:string)
                          n413 = local read "Test"() -> (w276:bool)
                          n414 = Concatenate Strings("%", w318, "\r\n", w309, w305, w308, "%\t\t", w304, w307, w303, w310) -> (w290:string)
                          n415 = Build Path(base path="Data Save Directory:", name or relative path=w282) -> (appended path=w289:path)
                          n416 = case shown="False" w276 {
                            tunnel: w290 -> [w325 _]
                            tunnel: w289 -> [w324 _]
                            tunnel: [w323 _] -> w288
                            tunnel: [w322 _] -> w286
                            frame False {
                              n417 = Write to Text File(file (use dialog)=w324, text=w325) -> (refnum out=w326:refnum<file>, error out=w327:errorcluster)  [unwired: 2 in, 1 out]
                              n418 = Close File(refnum=w326, error in=w327) -> (path=w323:path, error out=w322:errorcluster)
                            }
                            frame True {
                            }
                          }
                        }
                      }
                      n419 = Index Array(array="Visible Averages", index=3) -> (element=w224:bool)
                      n420 = Index Array(array="Visible Averages", index=1) -> (element=w225:bool)
                      n421 = Index Array(array="Visible Averages", index=0) -> (element=w218:bool)
                      n422 = Index Array(array="Visible Averages", index=2) -> (element=w219:bool)
                      n423 = property on="Tau 2" class="WFChart (strict)"("Active Plot"=u32 11) -> (error out=w222:errorcluster)  [unwired: 2 in, 1 out]
                      n424 = property on="Tau 2" class="WFChart (strict)"("Active Plot"=u32 9) -> (error out=w227:errorcluster)  [unwired: 2 in, 1 out]
                      n425 = property on="Tau 2" class="WFChart (strict)"("Active Plot"=u32 8) -> (error out=w216:errorcluster)  [unwired: 2 in, 1 out]
                      n426 = property on="Tau 2" class="WFChart (strict)"("Active Plot"=u32 10) -> (error out=w221:errorcluster)  [unwired: 2 in, 1 out]
                      n427 = property on="Tau 2" class="WFChart (strict)"(error in=w222, "Plot.Visible?"=w224) -> ()  [unwired: 1 in, 2 out]
                      n428 = property on="Tau 2" class="WFChart (strict)"(error in=w227, "Plot.Visible?"=w225) -> ()  [unwired: 1 in, 2 out]
                      n429 = property on="Tau 2" class="WFChart (strict)"(error in=w216, "Plot.Visible?"=w218) -> ()  [unwired: 1 in, 2 out]
                      n430 = property on="Tau 2" class="WFChart (strict)"(error in=w221, "Plot.Visible?"=w219) -> ()  [unwired: 1 in, 2 out]
                      n431 = local read "Test"() -> (w202:bool)
                      n432 = Not(x=w202) -> (.not. x?=w201:bool)
                      n433 = Unbundle By Name(w210) -> ("status"=w229:bool)
                      n434 = for {
                        N: 1 -> [_]
                        tunnel: w230 -> [_]
                        n435 = local write "Stop"(FALSE) -> ()
                        n436 = Wait (ms)(milliseconds to wait="Delay between frames(ms)") -> ()  [unwired: 1 out]
                      }
                      n437 = And(x="Real Time Fitting?", y=w201) -> (x .and. y?=w200:bool)
                      n438 = Not(x=w229) -> (.not. x?=w228:bool)
                      n439 = case shown="True" w200 {
                        tunnel: w228 -> [_ w239]
                        tunnel: w209 -> [_ w238]
                        tunnel: w208 -> [_ w237]
                        tunnel: w205 -> [w234 w236]
                        tunnel: [w234 w235] -> w204
                        frame False {
                        }
                        frame True {
                          n440 = case shown="True" w239 {
                            tunnel: w238 -> [_ w259]
                            tunnel: w237 -> [_ w255]
                            tunnel: w236 -> [w240 w251]
                            tunnel: [w240 w249] -> w235
                            frame False {
                            }
                            frame True {
                              # "Initialize Array of NaNs with size of \"fixed number of frames, \nand run this array into the case structure by putting it \nthrough a shift register with each loop it will replace one of \nthe NaNs by the flow data of the detector used. Then this data\nis averaged and COV is calculated."
                              n441 = property on="Data Save Directory:" class="Path"() -> ("Value"=w261:path)  [unwired: 2 in, 2 out]
                              n442 = property on="File Name (mouse#):" class="Str"() -> ("Value"=w262:string)  [unwired: 2 in, 2 out]
                              n443 = call "GetFilePath.vi"("path"=w261, "file name"=w262, "frame number"=w259) -> ("final path C"=w254:string)  [unwired: 10 in, 2 out]
                              n444 = property on="Avg" class="Arr (strict)"() -> ("Value"=w260:bool[][])  [unwired: 2 in, 2 out]
                              n445 = call "DCSAnalysis.vi"("# Detectors"=w255, "File path"=w254, "Frame #"=w259, "rho"="rho", "other settings"="Other Settings", "avgBool"=w260, "var values"="Initial Guess") -> ("Flow in each detector"=w252:dbl[], "Tau"=→"Tau 2":T3)  [unwired: 18 in, 1 out]
                              "Flow in each detector" <- w252
                              n446 = local read "Detector Used"() -> (w241:T2)
                              n447 = local read "Trial #"() -> (w247:u32)
                              n448 = Decrement(x=w247) -> (x-1=w248:u32)
                              n449 = Index Array(array=w252, index=w241) -> (element=w250:dbl)
                              n450 = Replace Array Subset(array=w251, new element=w250, index=w248) -> (w249:dbl[])
                              n451 = call <vilib>:"Std Deviation and Variance.vi"("X"=w249) -> ("mean"=w245:dbl, "standard deviation"=w246:dbl)  [unwired: 1 in, 1 out]
                              "mean" <- w245
                              n452 = Divide(x=w246, y=w245) -> (x/y=w243:dbl)
                              n453 = Multiply(x=w243, y=100.0) -> (x*y=→"COV":dbl)
                            }
                          }
                        }
                      }
                    }
                    n454 = call "iBs.vi"("Laser On/Off"=TRUE, "VISA resource name"="Laser Input Name") -> ()
                  }
                  frame True {
                    n455 = invoke on="Sequence Scan" class="Bool (strict)" method="Reinit To Default"() -> ()  [unwired: 3 in, 3 out]
                    n456 = call "Display Message to User5"() -> ()  [unwired: 10 in, 2 out]
                  }
                }
              }
            }
            "Frame #" <- u32 0
            "Mark #" <- u32 0
            "Trial #" <- u32 0
          }
          event "QUIT": Value Change {
            # "Reset correlator before quitting"
            n457 = event-data() -> ()  [unwired: 1 in, 6 out]
            n458 = case shown="\"8 Detectors\", Default" w637 {
              frame "4 Detectors" {
                n459 = dll-call lib="C:/Users/BUCKLEY-ADMIN/Desktop/GTcode_v6_Michelle/flex05-4chPascal.dll" fn="USBInitialize" label="InitCH4"() -> (error out=w639:errorcluster)  [unwired: 4 in, 1 out]
                n460 = dll-call lib="C:/Users/BUCKLEY-ADMIN/Desktop/GTcode_v6_Michelle/flex05-4chPascal.dll" fn="USBFree" label="FreeCH4"(error in=w639) -> ()  [unwired: 3 in, 2 out]
              }
              frame "8 Detectors", Default {
                n461 = dll-call lib="C:/Users/BUCKLEY-ADMIN/Desktop/GTcode_v6_Michelle/flex05oem8chauto100nsPASCAL_win7.dll" fn="USBInitialize" label="InitCH8"() -> (error out=w640:errorcluster)  [unwired: 4 in, 1 out]
                n462 = dll-call lib="C:/Users/BUCKLEY-ADMIN/Desktop/GTcode_v6_Michelle/flex05oem8chauto100nsPASCAL_win7.dll" fn="USBFree" label="FreeCH8"(error in=w640) -> ()  [unwired: 3 in, 2 out]
              }
            }
            n463 = local write "Status"("Quit") -> ()
            n464 = local write "Status"("Quit") -> ()
          }
          event Timeout {
            w645 = TRUE
            w644 = u8 0
            # "This case structure turns on\n      and off the ISS Lasers"
            # "This case structure ensures that when the\noptical switch is turned on, the relay tells \nthe laser to power on."
            # "The system sits here and wait for some buttons to be pressed. And the status is always \"waiting\". Once some button is pressed, this value driven event\nstructure goes to the appropriate frame."
            n465 = event-data() -> ()  [unwired: 1 in, 3 out]
            n466 = local write "Status"("Waiting") -> ()
            n467 = property on="MARK\nMark" class="Bool"("DisabledEnum"=w644) -> ()  [unwired: 2 in, 2 out]
            n468 = property on="QUIT" class="Bool"("Disabled"=w644) -> ()  [unwired: 2 in, 2 out]
            n469 = property on="Sequence Scan" class="Bool (strict)"("Disabled"=w644) -> ()  [unwired: 2 in, 2 out]
            n470 = property on="Initialize Correlator" class="Bool"("Disabled"=w644) -> ()  [unwired: 2 in, 2 out]
            n471 = property on="Update Time (ms)\nDO NOT CHANGE!" class="DigNum (strict)"("Disabled"=w644) -> ()  [unwired: 2 in, 2 out]
            n472 = property on="Integration Time (ms)" class="DigNum (strict)"("Disabled"=w644) -> ()  [unwired: 2 in, 2 out]
            n473 = property on="Detector Select" class="RadioBtnsControl (strict)"("Disabled"=w644) -> ()  [unwired: 2 in, 2 out]
            n474 = case shown="True" "ISS Lasers ON" {
              frame False {
                n475 = Build Array(FALSE) -> (w652:bool[])
                n476 = call "DAQ Assistant5"("data"=w652) -> ()  [unwired: 17 in, 2 out]
              }
              frame True {
                # "For Toptica laser control"
                n477 = local read "Laser Input Name"() -> (w654:refnum<visa-resource-name>)
                n478 = call "iBs.vi"("Laser On/Off"=TRUE, "VISA resource name"=w654) -> ()
                n479 = Build Array(TRUE) -> (w656:bool[])
                n480 = call "DAQ Assistant6"("data"=w656) -> ()  [unwired: 17 in, 2 out]
              }
            }
            n481 = case shown="True" "Optical Switch OPEN" {
              frame False {
                # "Send 2 signals, one for LED indicator, one for switch"
                n482 = Build Array(FALSE, FALSE) -> (w658:bool[])
                n483 = call "DAQ Assistant3"("data"=w658) -> ()  [unwired: 17 in, 2 out]
              }
              frame True {
                n484 = Build Array(TRUE, TRUE) -> (w661:bool[])
                n485 = call "DAQ Assistant4"("data"=w661) -> ()  [unwired: 17 in, 2 out]
              }
            }
            n486 = Current VI's Menubar() -> (w647:refnum<k9>)
            n487 = Set Menu Item Info(7:"File", 9:w645, 11:w647) -> (3:w646:refnum<k9>)  [unwired: 4 in, 1 out]
            n488 = Get Date/Time In Seconds() -> (seconds since 1Jan1904=w650:timestamp)
            n489 = Set Menu Item Info(7:"Options", 9:w645, 11:w646) -> ()  [unwired: 4 in, 2 out]
            n490 = Format Date/Time String(seconds (now)=w650) -> (date/time string=w651:string)  [unwired: 2 in]
            n491 = local write "Computer Time"(w651) -> ()
          }
        }
      }
    }
  }
